vi "main.vi"(0 "Test Pins":T6, 1 "Caller Information":T7, 5 "Test Inputs":T10={"Load Current 1 in A"=0.0, "Load Current 2 in A"=0.0, "Duration of the pulse in Second"=0.5, "Nominal Output Voltage in V"=0.0, "Ref Voltage level for Settling Time Calc"=0.1, "% of Vnom for Settling Time Calc"=10.0, "Settling Time Calc Option"=enum."Voltage Level ", "Advance Setting"={"Prepare"={"Load SMU Record Length"=2}}, "Save Transient Graph?"=TRUE, "Input Voltage in V"=0.0, "Save Scope Raw Data?"=FALSE, "Delay - t1 in s"=0.25, "Delay - t2 in s"=0.25, "Auto Scale Y-Axis?"=TRUE, "Shunt Resistance (Ohm)"=1.0}, 11 "error in":errorcluster) -> (4 "Test Results":T14 {"Second Edge - Settling Time in s" format="%#.5p"; "First Edge - Settling Time in s" format="%#.5p"; "Actual Sample Rate in S/s" format="%#.5g"}, 15 "error out":errorcluster)   [LabVIEW 2020, in "LDO Load Transient.lvlib"]
doc: "<b>Caller</b> Information is input for framework components. Mode should be set to <b>Automation</b> when running from TestStand. Sequence Context should be set to <b>ThisContext</b> when running from TestStand. The values will be updated everytime the setting is applied using \"Edit\" dialog.\n\n<b>Test Pins</b> is names of pins available in the pinmap file. Provide the right pins for the required functionality.\n\n<b>Test Inputs</b> is input required for the measurement to perform.\n\n<b>error in</b> is meant for the sequencing. <b>error in</b> should be <b>no error</b> always.\n\n<b>Test Results</b> contains all the measured data during the measurement and processed results.\n\n<b>error out</b> contains the error occured during measurement.\n\nCheck measurement documentation for more information (<Program Files>\\Soliton Technologies\\MeasurementSuite\\CodeModules\\LDO\\LDO Load Transient.pdf)"
uses:
  LDO Load Transient.lvlib
  Typedefs/Test Results.ctl
  Typedefs/Test Inputs.ctl
  Typedefs/Settling Time Calc Option.ctl
  Typedefs/Advance Settings.ctl
  Typedefs/Adv Settings Setup Instr.ctl
  <userlib>/_Soliton/Measurement Suite/Reusables/Plugin Common/Typedefs/Caller Events.ctl
  <userlib>/_Soliton/Measurement Suite/Reusables/Plugin Common/Typedefs/Caller Information.ctl
  <userlib>/_Soliton/Measurement Suite/Reusables/Plugin Common/Typedefs/Caller Mode.ctl
  Typedefs/Test Pins.ctl
  Typedefs/Pin Dropdown.ctl
  <userlib>/_Soliton/Measurement Suite/Reusables/Plugin Common/Typedefs/Termination Monitor Info.ctl
  Typedefs/Current Measurement Type.ctl
  Reusables/UI/Progress Monitor/Progress Monitor Option.ctl
  <vilib>/Utility/miscctls.llb/LVMajorAndMinorColorsTypeDef.ctl
  <instrlib>/niDCPower/nidcpower.llb/niDCPower Source Mode.ctl
  <instrlib>/niDCPower/nidcpower.llb/niDCPower Output Function.ctl
  <instrlib>/niDCPower/nidcpower.llb/niDCPower Wait For Event - Event.ctl
  <vilib>/Utility/error.llb/DialogType.ctl
  63a61bec-041e-4365-831b-8165c1c311c6.vi
  d648f1df-a8d9-4085-9eb0-24252e83c66e.vi
  98c31a9a-65c4-404a-8d29-5fef3c3d30dc.vi
  feeae9f6-ae23-4438-849e-34acdc15b747.vi
  e89c743e-5273-4ded-a4f4-1d44fefc8133.vi
  44f97677-0516-4608-8e28-d738a12fef77.vi
  01e50ca5-2bbf-454e-9d2d-d5f5dbc62a55.vi
  49732470-67c5-4264-8b59-91d7a6bf13ef.vi
  29f2f23f-c0b0-483c-8177-98a50cbfcdf1.vi
  bb3e62c4-a2c2-4505-9438-f842dd651d6c.vi
  ce2ee1e5-697c-4608-b941-8c9b0f21ffd9.vi
  217e438d-a1ad-49ce-9dcd-d015b5ab8206.vi
  3210b59a-1980-40a2-8b26-190a43568d65.vi
  <userlib>/_Soliton/Measurement Suite/Reusables/InstrumentSessionAPIs/SessionManagerApiPath.vi
  <vilib>/Utility/sysdir.llb/Get System Directory.vi
  <vilib>/Utility/LVLibp/Get Exported File Path.vi
  <userlib>/_Soliton/Measurement Suite/Reusables/Errors/Error 6001.vi
  <userlib>/_Soliton/Measurement Suite/Reusables/Plugin Common/Plugin Common.lvlib
  <userlib>/_Soliton/Measurement Suite/Reusables/Queue Driver/Plugin Queue Driver.lvlib
panel:
  out "Progress":i32(slide) scale=-1.0..17.0
  in  "Terminate":bool
  in  "Run":bool caption="Measure"
  in  "Exit":bool
  out "Header":string
  in  "Tab Enum":T1(radio)
  out "Tab Control":T2(tab)
  in  "Shunt Resistance (Ohm)":dbl=1.0 min=1.0 format="%#_6p"
  in  "SystemSetup":T4={"Set Load Current"={"PinStatus"=0, "PinName"="", "Info"=TRUE}, "Set Input Voltage"={"PinStatus"=0, "PinName"="", "Info"=TRUE}, "Measure Output Voltage"={"PinStatus"=0, "PinName"="", "Info"=TRUE}, "Measure Load Current"={"PinStatus"=0, "PinName"="", "Info"=TRUE}}
  out "Shunt Resistance Info":u16(ring) caption="Set 1 Ohm if its Current Probe"
  out "Sequence Timeout":dbl caption="Sequence Timeout (s)" format="%#.5p"
  in  "Delay - t2 (s)":dbl=0.25 format="%#_6p"
  in  "Delay - t1 (s)":dbl=0.25 format="%#_6p"
  in  "Duration of the pulse (s)":dbl=0.5 format="%#_6p"
  in  "Percentage of Vnom (%)":dbl=10.0 caption="Percentage of nominal voltage (%)" format="%#_6f"
  in  "Voltage to settle above Vnom (V)":dbl=0.1 format="%#_6p"
  in  "Load Current 1 - Iload1 (A)":dbl format="%#_6p"
  in  "Settling Time Calculation":enum32{"Item 0", "Item 1"}(radio)
  in  "Input Voltage (V)":dbl format="%#_6p"
  in  "Load Current 2 - Iload2 (A)":dbl format="%#_6p"
  in  "Nominal Output Voltage (V)":dbl format="%#_6p"
  in  "Advanced Settings":bool
  out "Second Edge - Settling Time (s)":dbl format="%#.5p"
  in  "Auto Scale Y-Axis?":bool=TRUE
  in  "Save Scope Raw Data?":bool=TRUE
  out "Load Transient":cluster{"x-axis":dbl[], "wfm":dbl[]}[](graph)
  in  "Take Transient snapshot?":bool=TRUE
  out "Transient Load Current":waveform(dbl)(graph)
  out "Transient Output Voltage":T5(graph)
  out "First Edge - Settling Time (s)":dbl format="%#.5p"
  in  "Caller Events":T9
  in  "DataLogPath":path
  in  "ErrorOccured":errorcluster
  # "Supports NIDCPowerInstrument"
  # "Supports NIScopeInstrument"
  # "Supports NIDCPowerInstrument"
  # "Supports NIScopeInstrument,NIDCPowerInstrument"
  # "Load Current"
  # "Minimum value for Delay-t1, Duration of the pulse, Delay-t2 should be larger than [ ( Souredelay+Aperture Time ) x Record Length ]"
  # "Settling Time Calculation"
  # "Settling Time is defined as the time taken for the output voltage to recover\nto the LDO nominal output voltage."
  # "Time taken for output voltage to settle to (Choose one below)"
  # "Load Transient"
  # "Output Voltage"
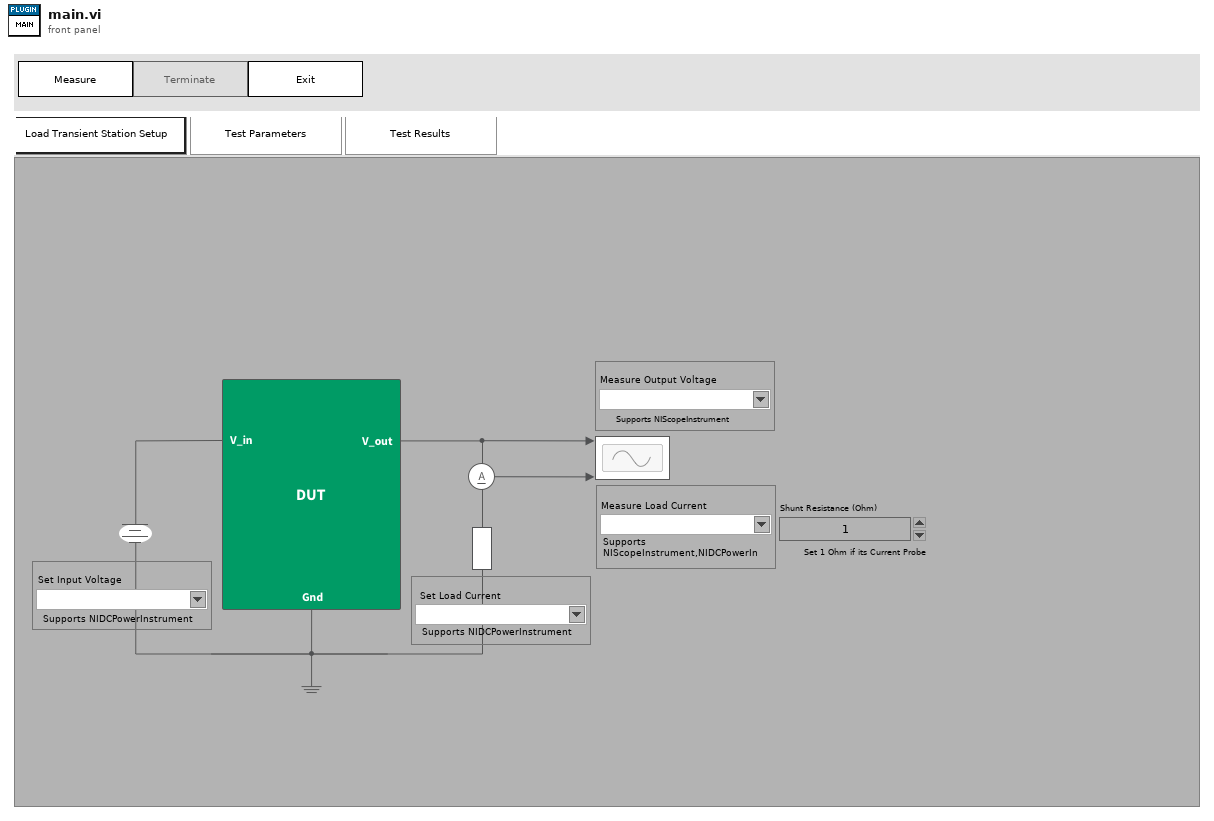
[diagram p1: front panel]
types:
  T1 = enum32{"Station Setup", "Test Parameters", "Test Results"}
  T2 = enum32{"Station Setup", "Test Parameters", "Test Results", "Debug"}
  T3 = typedef "LDO Load Transient.lvlib/Pin Dropdown.ctl" = cluster{"PinStatus":u16, "PinName":string, "Info":bool}
  T4 = cluster{"Set Load Current":T3, "Set Input Voltage":T3, "Measure Output Voltage":T3, "Measure Load Current":T3}
  T5 = cluster{"relativeInitialX":dbl, "xIncrement":dbl, "wfm":dbl[]}
  T6 = typedef "LDO Load Transient.lvlib/Test Pins.ctl" = cluster{"Set Input Voltage":string, "Set Load Current":string, "Measure Output Voltage":string, "Measure Load Current":string}
  T7 = typedef "Plugin Common.lvlib/Caller Information.ctl" = cluster{"Mode":T8, "Sequence Context":refnum<k7>}
  T8 = typedef "Caller Mode.ctl" = enum16{"Standalone", "Automation", "MeasurementSuite"}
  T9 = typedef "Plugin Common.lvlib/Caller Events.ctl" = cluster{"Caller Event":refnum<user-event>}
  T10 = typedef "LDO Load Transient.lvlib/Test Inputs.ctl" = cluster{"Load Current 1 in A":dbl, "Load Current 2 in A":dbl, "Duration of the pulse in Second":dbl, "Nominal Output Voltage in V":dbl, "Ref Voltage level for Settling Time Calc":dbl, "% of Vnom for Settling Time Calc":dbl, "Settling Time Calc Option":T11, "Advance Setting":T12, "Save Transient Graph?":bool, "Input Voltage in V":dbl, "Save Scope Raw Data?":bool, "Delay - t1 in s":dbl, "Delay - t2 in s":dbl, "Auto Scale Y-Axis?":bool, "Shunt Resistance (Ohm)":dbl}
  T11 = typedef "LDO Load Transient.lvlib/Settling Time Calc Option.ctl" = enum16{"Voltage Level ", "Percentage of Vnom"}
  T12 = typedef "LDO Load Transient.lvlib/Advance Settings.ctl" = cluster{"Prepare":T13}
  T13 = typedef "LDO Load Transient.lvlib/Adv Settings Setup Instr.ctl" = cluster{"Load SMU Record Length":i32}
  T14 = typedef "LDO Load Transient.lvlib/Test Results.ctl" = cluster{"Measured Output Voltage":cluster{"x-axis":dbl[], "wfm":dbl[]}, "Measured Load Current":cluster{"x-axis":dbl[], "wfm":dbl[]}, "Actual Sample Rate in S/s":dbl, "First Edge - Settling Time in s":dbl, "Second Edge - Settling Time in s":dbl}
  T15 = typedef "Plugin Common.lvlib/Termination Monitor Info.ctl" = cluster{"Caller Information":T7, "Execution":refnum<k7>, "Termination Monitor":refnum<k7>, "Type":string, "Plugin Name":string}
  T16 = typedef "LDO Load Transient.lvlib/Current Measurement Type.ctl" = enum16{"Scope Measurement", "SMU Measurement"}
  T17 = cluster{"Termination Monitor Info":T15, "Test Inputs":T10, "Test Results":T14, "Test Results[][]":string[][], "Test Pins":T6, "Logger Folder Path":path, "Valid Logger Path?":bool, "Logger File Path":path, "Load Current Waveform":dbl[], "Load Current Source Delay":dbl[], "Min delay for Reference Position":u32, "Output Voltage Coupling":i32, "Current Measurement Option":T16, "Sequence name":string, "UI Ctls":refnum<vi>[], "Insufficient memory?":bool, "Scope Record Length":i32, "Scope Channels":string, "Sequence Empty?":bool}
  T18 = typedef "Progress Monitor Option.ctl" = enum16{"State Array Init", "Get State Index"}
  T19 = enum8{"Enabled", "Disabled", "Disabled and Grayed Out"}
  T20 = cluster{"Set Iload":T3, "Set Vin":T3, "Capture Output Voltage":T3, "Capture Output Current":T3}
  T21 = typedef "LVMajorAndMinorColorsTypeDef.ctl" = cluster{"Major Color":u32, "Minor Color":u32}
  T22 = typedef "niDCPower Wait For Event - Event.ctl" = i32
  T23 = typedef "niDCPower Output Function.ctl" = i32
  T24 = typedef "niDCPower Source Mode.ctl" = i32
  T25 = typedef "DialogType.ctl" = u16
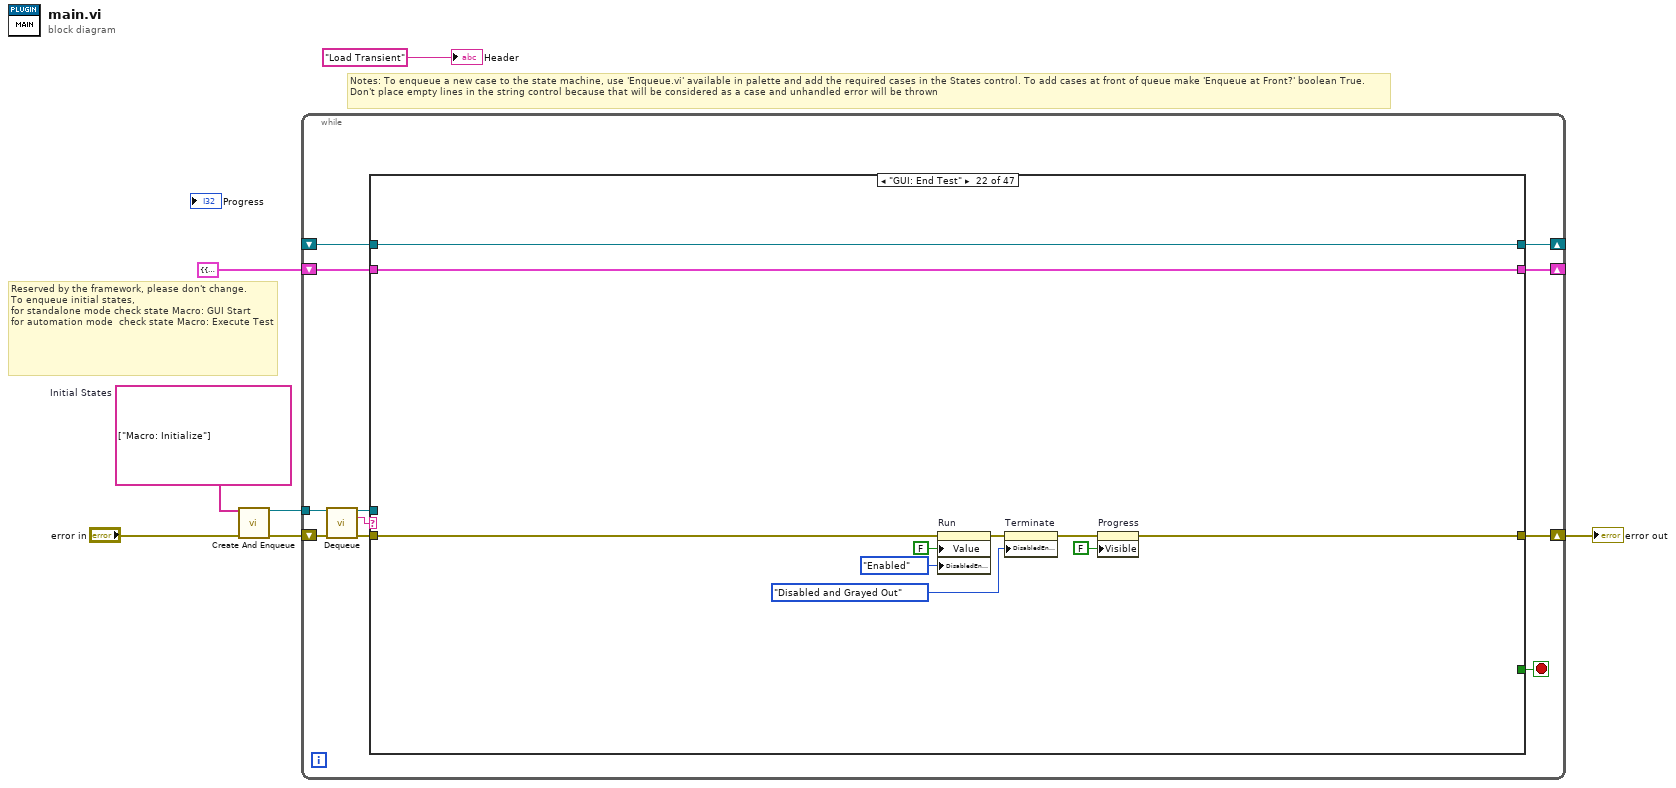
[diagram p0: block diagram]
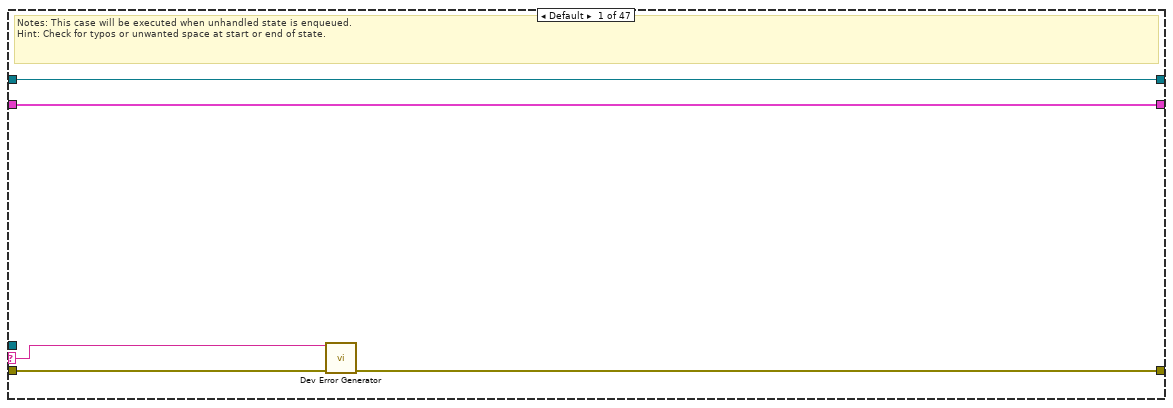
[diagram p2: hidden frame]
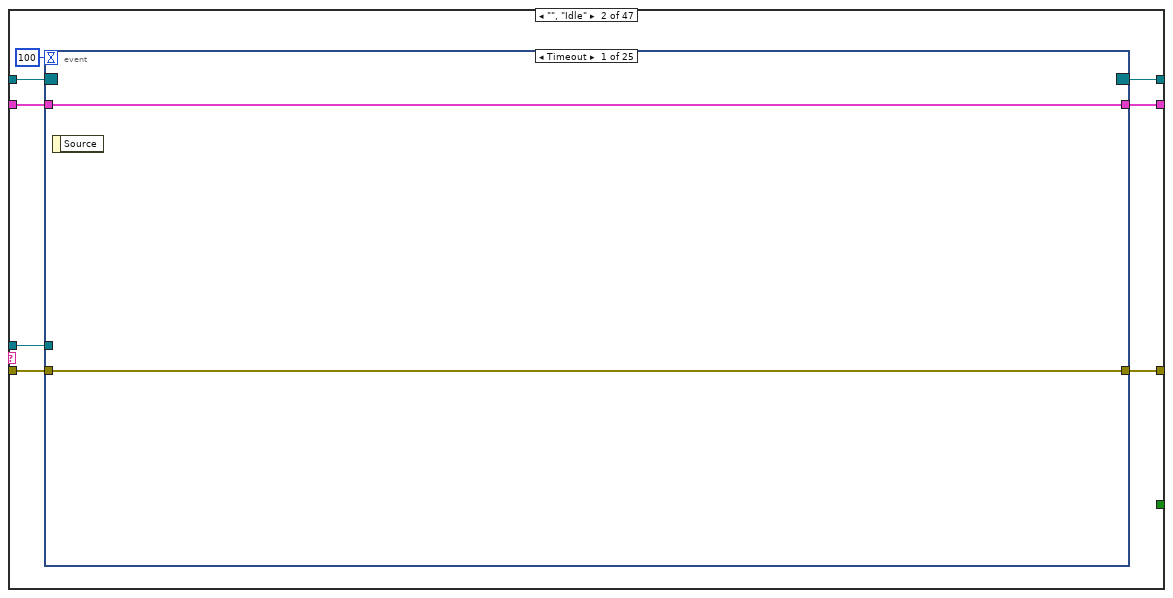
[diagram p3: hidden frame]
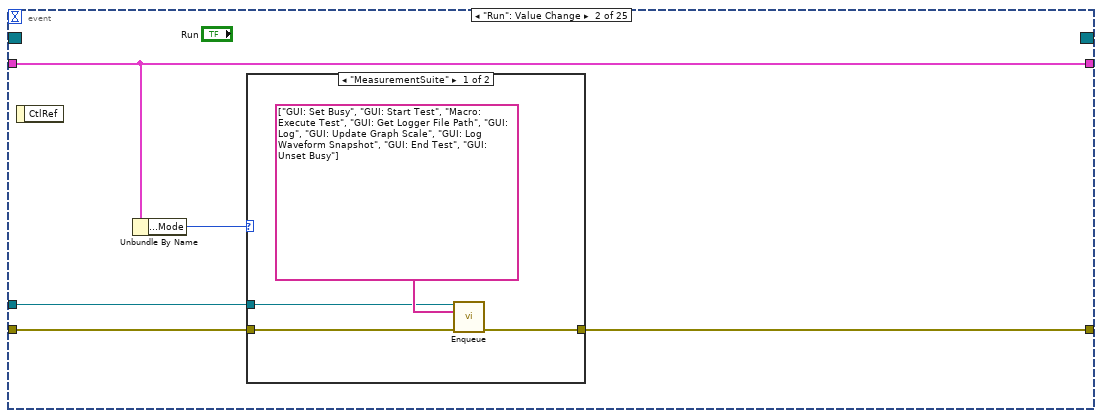
[diagram p4: hidden frame]
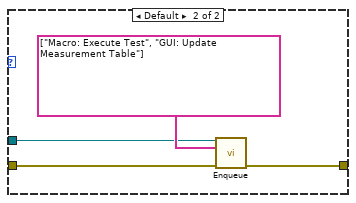
[diagram p5: hidden frame]
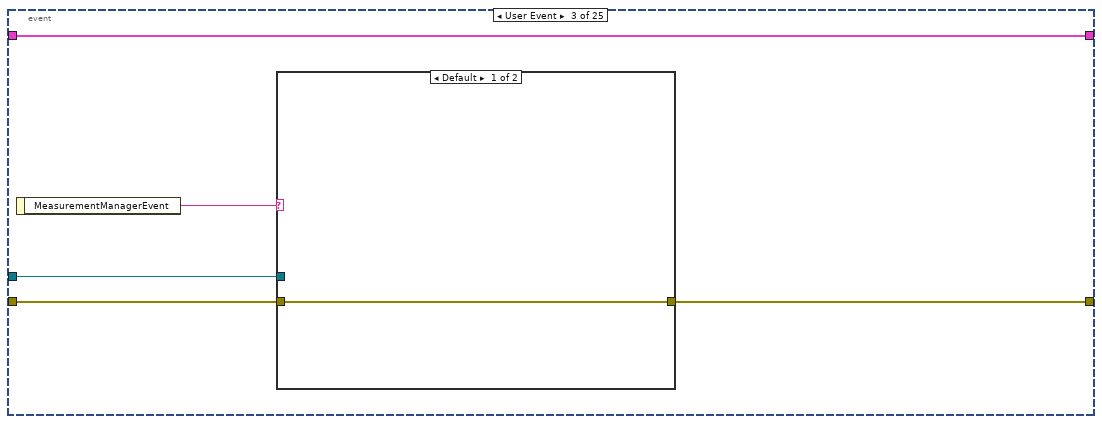
[diagram p6: hidden frame]
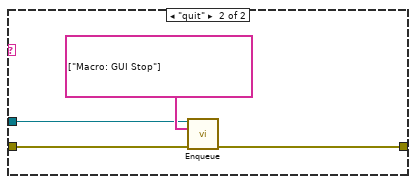
[diagram p7: hidden frame]
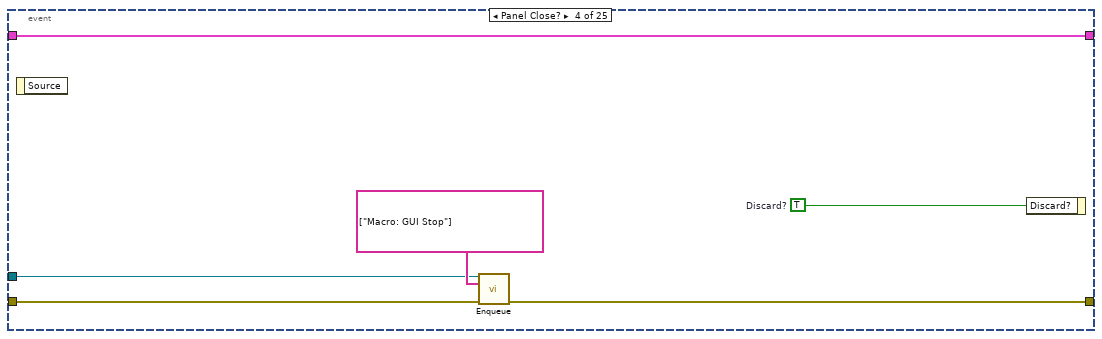
[diagram p8: hidden frame]
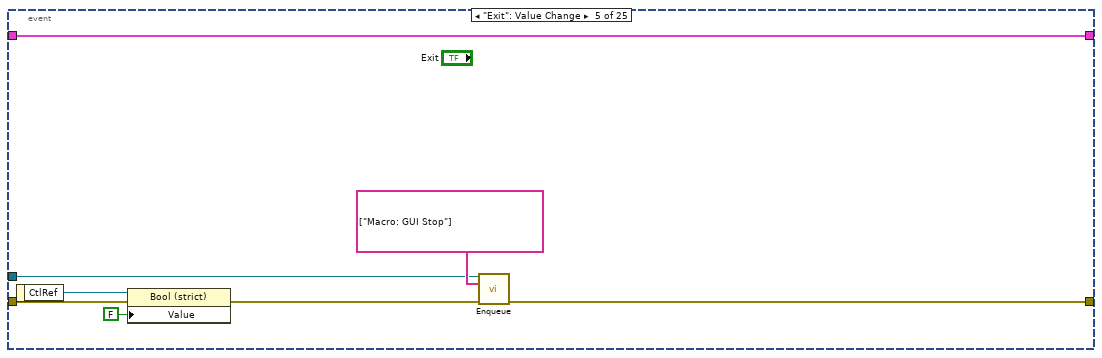
[diagram p9: hidden frame]
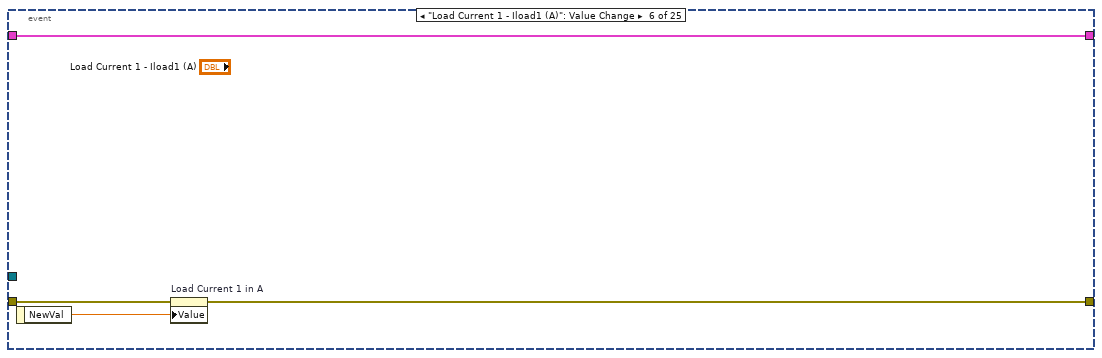
[diagram p10: hidden frame]
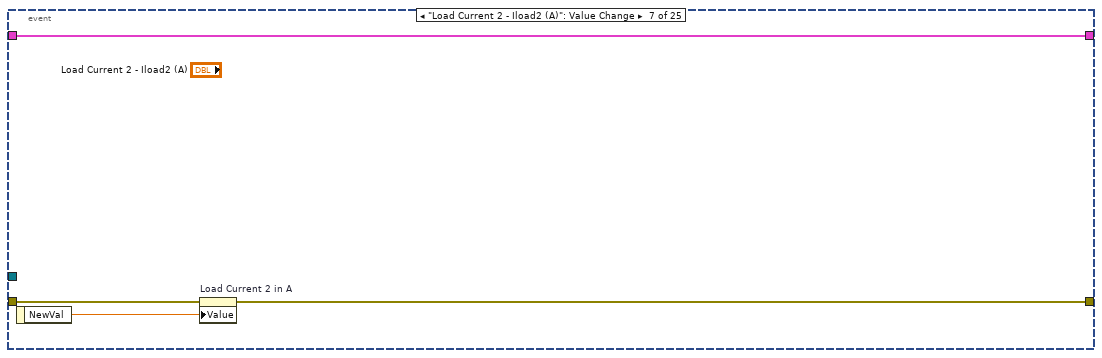
[diagram p11: hidden frame]
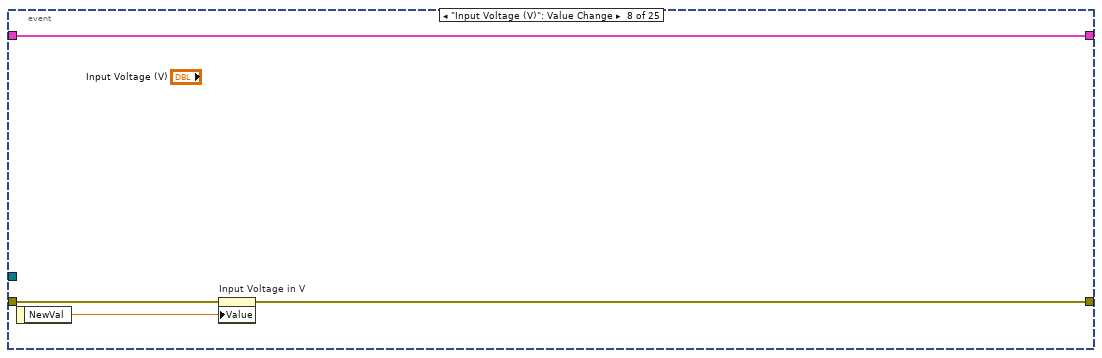
[diagram p12: hidden frame]
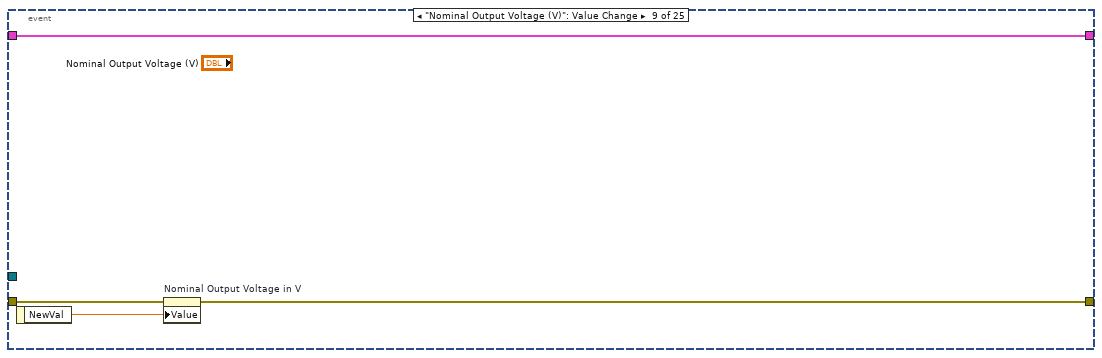
[diagram p13: hidden frame]
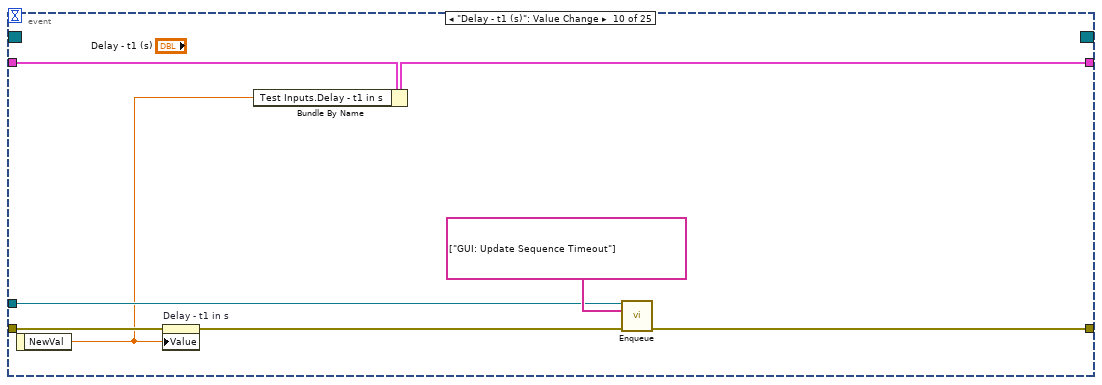
[diagram p14: hidden frame]
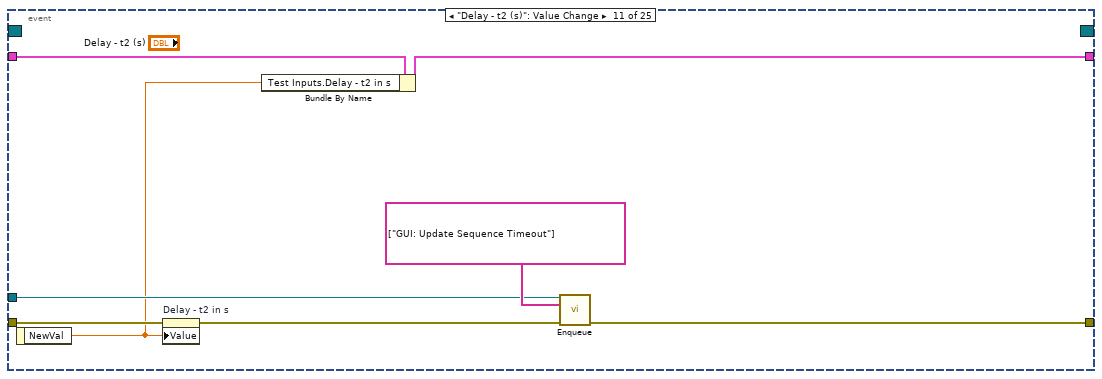
[diagram p15: hidden frame]
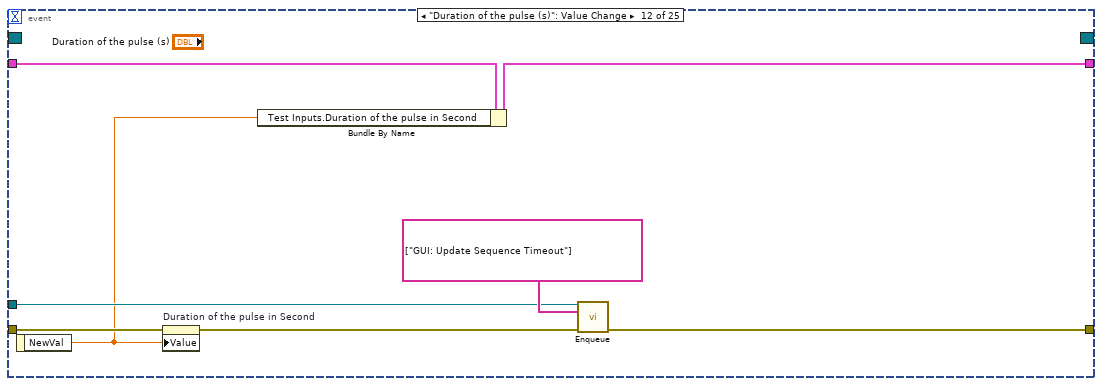
[diagram p16: hidden frame]
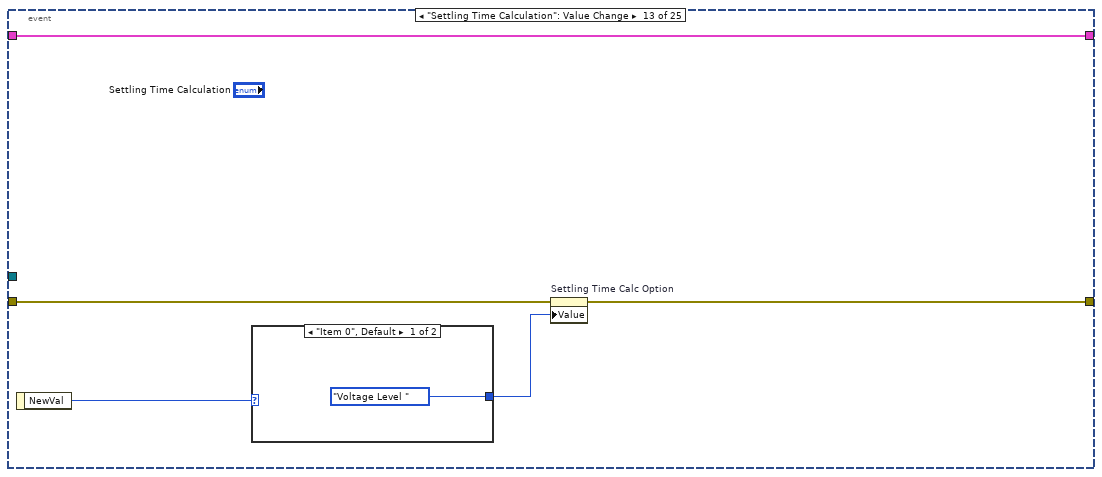
[diagram p17: hidden frame]
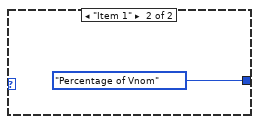
[diagram p18: hidden frame]
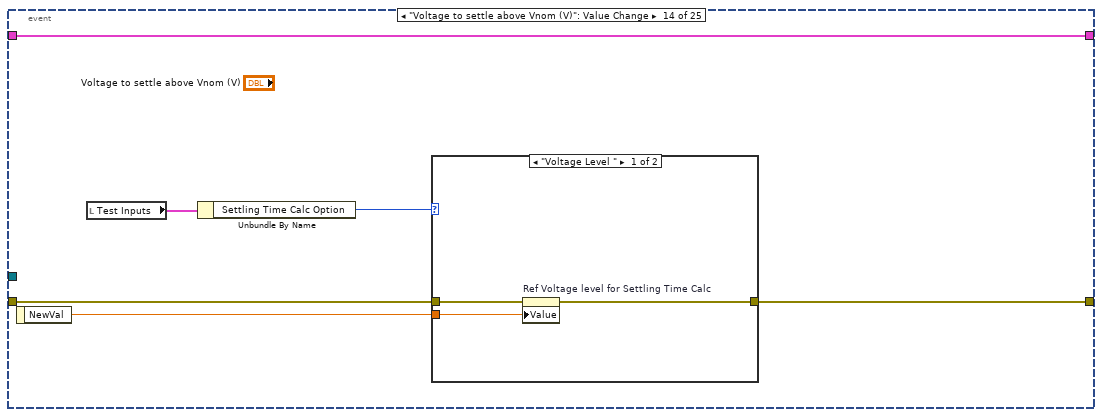
[diagram p19: hidden frame]
diagram:
  w7 = string[] ["Macro: Initialize"]  # Initial States
  # "Notes: To enqueue a new case to the state machine, use 'Enqueue.vi' available in palette and add the required cases in the States control. To add cases at front of queue make 'Enqueue at Front?' boolean True. Don't place empty lines in the string control because that will be considered as a case and unhandled error will be thrown"
  # "Reserved by the framework, please don't change. \nTo enqueue initial states,\nfor standalone mode check state Macro: GUI Start\nfor automation mode  check state Macro: Execute Test"
  n1 = call <userlib>:"Create And Enqueue.vi"("Initial States"=w7, "error in (no error)"="error in") -> ("Queue out"=w5:refnum<queue>, "error out"=w3:errorcluster)  [unwired: 12 in]
  n2 = while {
    shift-right: [w18] -> w4
    shift-left: w3 -> [w16]
    shift-right: [w14] -> _
    shift-left: T17 {"Termination Monitor Info"={"Caller Information"={"Mode"=enum."Standalone", "Sequence Context"=refnum}, "Execution"=refnum, "Termination Monitor"=refnum, "Type"="", "Plugin Name"=""}, "Test Inputs"={"Load Current 1 in A"=0.0, "Load Current 2 in A"=0.0, "Duration of the pulse in Second"=0.0, "Nominal Output Voltage in V"=0.0, "Ref Voltage level for Settling Time Calc"=0.0, "% of Vnom for Settling Time Calc"=0.0, "Settling Time Calc Option"=enum."Voltage Level ", "Advance Setting"={"Prepare"={"Load SMU Record Length"=0}}, "Save Transient Graph?"=FALSE, "Input Voltage in V"=0.0, "Save Scope Raw Data?"=FALSE, "Delay - t1 in s"=0.0, "Delay - t2 in s"=0.0, "Auto Scale Y-Axis?"=FALSE, "Shunt Resistance (Ohm)"=0.0}, "Test Results"={"Measured Output Voltage"={"x-axis"=[], "wfm"=[]}, "Measured Load Current"={"x-axis"=[], "wfm"=[]}, "Actual Sample Rate in S/s"=0.0, "First Edge - Settling Time in s"=0.0, "Second Edge - Settling Time in s"=0.0}, "Test Results[][]"=[], "Test Pins"={"Set Input Voltage"="", "Set Load Current"="", "Measure Output Voltage"="", "Measure Load Current"=""}, "Logger Folder Path"=path "", "Valid Logger Path?"=FALSE, "Logger File Path"=path "", "Load Current Waveform"=[], "Load Current Source Delay"=[], "Min delay for Reference Position"=0, "Output Voltage Coupling"=0, "Current Measurement Option"=enum."Scope Measurement", "Sequence name"="CurrentSequence", "UI Ctls"=[], "Insufficient memory?"=FALSE, "Scope Record Length"=0, "Scope Channels"="", "Sequence Empty?"=TRUE} -> [w13]
    tunnel: w5 -> [w12]
    shift-right: [w9] -> _
    shift-left: _ -> [w10]
    stop <- w17 stop-if-true
    n3 = call <userlib>:"Dequeue.vi"("Queue in"=w12, "error in (no error)"=w16) -> ("Queue out"=w11:refnum<queue>, "Dequeued State"=w8:string, "error out"=w15:errorcluster)  [unwired: 11 in]
    n4 = case shown="\"GUI: End Test\"" w8 {
      selector: w8 -> [w21 _ _ _ _ _ _ _ _ _ _ _ w345 w361 _ _ _ _ _ _ _ _ _ _ _ _ w537 w554 w567 w602 w630 w675 _ _ w746 w755 w795 w834 w867 w883 w928 w955 w981 w990 _ _ _]
      tunnel: w15 -> [w20 w28 w251 w260 w275 w281 w288 w293 w326 w337 w341 w344 w346 w363 w378 w391 w403 w432 w445 w466 w498 w507 w518 w523 w530 w535 w538 w555 w568 w603 w631 w676 w692 w706 w747 w756 w796 w835 w868 w884 w929 w956 w982 w991 w998 w1005 w1023]
      tunnel: [w22 w29 w251 w263 w266 w282 w289 w293 w324 w335 w339 w344 w350 w366 w379 w392 w402 w433 w443 w467 w499 w506 w518 w524 w531 w535 w544 w561 w566 w584 w634 w683 w693 w707 w745 w763 w790 w829 w869 w885 w915 w959 w983 w992 w998 w1003 w1017] -> w18
      tunnel: [_ _ _ _ _ _ _ _ _ _ _ _ _ _ _ _ _ _ _ _ _ _ _ _ _ _ _ _ _ _ _ _ _ _ _ _ _ _ _ _ _ _ _ _ _ w1000 TRUE] -> w17
      tunnel: [w23 w31 w250 w253 w276 w283 w290 w292 w315 w336 w340 w343 w349 w365 w380 w398 w401 w434 w459 w465 w505 w515 w517 w522 w529 w534 w543 w560 w571 w608 w629 w681 w691 w709 w750 w760 w798 w838 w872 w888 w936 w961 w988 w995 w997 w1002 w1024] -> w14
      tunnel: w13 -> [w23 w30 w250 w264 w276 w283 w290 w292 w331 w336 w340 w343 w349 w365 w380 w398 w400 w434 w459 w465 w505 w515 w517 w521 w528 w534 w553 w559 w571 w608 w628 w680 w690 w708 w750 w759 w798 w837 w871 w887 w936 w961 w988 w995 w997 w1002 w1024]
      tunnel: w11 -> [_ w24 _ w262 w274 w279 w286 _ _ _ _ _ _ _ _ _ _ _ _ _ _ _ _ _ _ _ _ _ _ _ _ _ _ _ _ _ _ _ _ _ _ _ _ _ _ w999 w1022]
      tunnel: w10 -> [w19 w26 w249 w261 w273 w278 w285 w291 w330 _ w338 w342 w356 w372 w381 w399 w408 w435 w460 w472 w504 w514 w516 w525 w532 w533 w551 w563 w572 w609 w636 w688 w695 w711 w751 w764 w799 w839 w878 w897 w937 w966 w989 w994 w996 w1004 w1021]
      tunnel: [w19 w25 w249 w261 w273 w278 w285 w291 w330 w334 w338 w342 w356 w372 w381 w399 w408 w435 w460 w472 w504 w514 w516 w525 w532 w533 w551 w563 w572 w609 w636 w688 w695 w711 w751 w764 w799 w839 w878 w897 w937 w966 w989 w994 w996 w1004 w1021] -> w9
      frame Default {
        # "Notes: This case will be executed when unhandled state is enqueued. \nHint: Check for typos or unwanted space at start or end of state."
        n5 = call <userlib>:"Dev Error Generator.vi"("State"=w21, "error in (no error)"=w20) -> ("error out"=w22:errorcluster)  [unwired: 13 in]
      }
      frame "", "Idle" {
        n6 = event shown="[0] Timeout" {
          selector: w26 -> [_ _ _ _ _ _ _ _ _ _ _ _ _ _ _ _ _ _ _ _ _ _ _ _ _]
          dyn-events: [_ _ _ _ _ _ _ _ _ _ _ _ _ _ _ _ _ _ _ _ _ _ _ _ _] -> w25
          timeout: 100 -> [_ _ _ _ _ _ _ _ _ _ _ _ _ _ _ _ _ _ _ _ _ _ _ _ _]
          tunnel: [w33 w35 w51 w62 w70 w74 w78 w82 w86 w89 w97 w105 w115 w123 w134 w145 w149 w153 w158 w169 w188 w232 w237 w242 w248] -> w31
          tunnel: w30 -> [w33 w35 w51 w62 w70 w74 w78 w82 w86 w88 w96 w104 w115 w123 w134 w145 w149 w153 w160 w168 w187 w231 w237 w241 w248]
          tunnel: [w32 w38 w49 w59 w68 w73 w77 w80 w85 w91 w99 w107 w112 w121 w131 w143 w147 w151 w154 w167 w179 w213 w236 w239 w246] -> w29
          tunnel: w28 -> [w32 w37 w50 w58 w67 w72 w76 w81 w84 w94 w102 w110 w113 w122 w130 w144 w148 w152 w159 w170 w190 w212 w236 w244 w247]
          tunnel: w24 -> [_ w36 w47 w57 w66 _ _ _ _ w90 w98 w106 _ _ _ _ _ _ _ w166 w178 _ _ _ _]
          event Timeout {
            n7 = event-data() -> ()  [unwired: 1 in, 1 out]
          }
          event "Run": Value Change {
            n8 = event-data() -> ()  [unwired: 1 in, 1 out]
            n9 = Unbundle By Name(w35) -> ("Termination Monitor Info.Caller Information.Mode"=w34:T8)
            n10 = case shown="\"MeasurementSuite\"" w34 {
              tunnel: [w41 w45] -> w38
              tunnel: w37 -> [w40 w44]
              tunnel: w36 -> [w39 w43]
              frame "MeasurementSuite" {
                n11 = call <userlib>:"Enqueue.vi"("Queue in"=w39, "States"=string[] ["GUI: Set Busy", "GUI: Start Test", "Macro: Execute Test", "GUI: Get Logger File Path", "GUI: Log", "GUI: Update Graph Scale", "GUI: Log Waveform Snapshot", "GUI: End Test", "GUI: Unset Busy"], "error in (no error)"=w40) -> ("error out"=w41:errorcluster)  [unwired: 11 in, 1 out]
              }
              frame Default {
                n12 = call <userlib>:"Enqueue.vi"("Queue in"=w43, "States"=string[] ["Macro: Execute Test", "GUI: Update Measurement Table"], "error in (no error)"=w44) -> ("error out"=w45:errorcluster)  [unwired: 11 in, 1 out]
              }
            }
          }
          event User Event {
            n13 = event-data() -> ("MeasurementManagerEvent"=w48:string)  [unwired: 1 in]
            n14 = case shown="Default" w48 {
              tunnel: [w52 w53] -> w49
              tunnel: w50 -> [w52 w55]
              tunnel: w47 -> [_ w54]
              frame Default {
              }
              frame "quit" {
                n15 = call <userlib>:"Enqueue.vi"("Queue in"=w54, "States"=string[] ["Macro: GUI Stop"], "error in (no error)"=w55) -> ("error out"=w53:errorcluster)  [unwired: 11 in, 1 out]
              }
            }
          }
          event Panel Close? {
            w61 = TRUE  # Discard?
            n16 = event-data() -> ()  [unwired: 1 in, 1 out]
            n17 = call <userlib>:"Enqueue.vi"("Queue in"=w57, "States"=string[] ["Macro: GUI Stop"], "error in (no error)"=w58) -> ("error out"=w59:errorcluster)  [unwired: 11 in, 1 out]
            n18 = event-data("Discard?"=w61) -> ()  [unwired: 1 in, 1 out]
          }
          event "Exit": Value Change {
            n19 = event-data() -> ("CtlRef"=w64:refnum<vi>)  [unwired: 1 in]
            n20 = property class="Bool (strict)"(reference=w64, error in=w67, "Value"=FALSE) -> (error out=w65:errorcluster)  [unwired: 1 out]
            n21 = call <userlib>:"Enqueue.vi"("Queue in"=w66, "States"=string[] ["Macro: GUI Stop"], "error in (no error)"=w65) -> ("error out"=w68:errorcluster)  [unwired: 11 in, 1 out]
          }
          event "Load Current 1 - Iload1 (A)": Value Change {
            n22 = event-data() -> ("NewVal"=w71:dbl)  [unwired: 1 in]
            n23 = property on="Load Current 1 in A" class="DigNum (strict)"(error in=w72, "Value"=w71) -> (error out=w73:errorcluster)  [unwired: 1 in, 1 out]
          }
          event "Load Current 2 - Iload2 (A)": Value Change {
            n24 = event-data() -> ("NewVal"=w75:dbl)  [unwired: 1 in]
            n25 = property on="Load Current 2 in A" class="DigNum (strict)"(error in=w76, "Value"=w75) -> (error out=w77:errorcluster)  [unwired: 1 in, 1 out]
          }
          event "Input Voltage (V)": Value Change {
            n26 = event-data() -> ("NewVal"=w79:dbl)  [unwired: 1 in]
            n27 = property on="Input Voltage in V" class="DigNum (strict)"(error in=w81, "Value"=w79) -> (error out=w80:errorcluster)  [unwired: 1 in, 1 out]
          }
          event "Nominal Output Voltage (V)": Value Change {
            n28 = event-data() -> ("NewVal"=w83:dbl)  [unwired: 1 in]
            n29 = property on="Nominal Output Voltage in V" class="DigNum (strict)"(error in=w84, "Value"=w83) -> (error out=w85:errorcluster)  [unwired: 1 in, 1 out]
          }
          event "Delay - t1 (s)": Value Change {
            n30 = event-data() -> ("NewVal"=w87:dbl)  [unwired: 1 in]
            n31 = property on="Delay - t1 in s" class="DigNum (strict)"(error in=w94, "Value"=w87) -> (error out=w92:errorcluster)  [unwired: 1 in, 1 out]
            n32 = Bundle By Name(cluster=w88, "Test Inputs.Delay - t1 in s"=w87) -> (w89:T17)
            n33 = call <userlib>:"Enqueue.vi"("Queue in"=w90, "States"=string[] ["GUI: Update Sequence Timeout"], "error in (no error)"=w92) -> ("error out"=w91:errorcluster)  [unwired: 11 in, 1 out]
          }
          event "Delay - t2 (s)": Value Change {
            n34 = event-data() -> ("NewVal"=w95:dbl)  [unwired: 1 in]
            n35 = property on="Delay - t2 in s" class="DigNum (strict)"(error in=w102, "Value"=w95) -> (error out=w100:errorcluster)  [unwired: 1 in, 1 out]
            n36 = Bundle By Name(cluster=w96, "Test Inputs.Delay - t2 in s"=w95) -> (w97:T17)
            n37 = call <userlib>:"Enqueue.vi"("Queue in"=w98, "States"=string[] ["GUI: Update Sequence Timeout"], "error in (no error)"=w100) -> ("error out"=w99:errorcluster)  [unwired: 11 in, 1 out]
          }
          event "Duration of the pulse (s)": Value Change {
            n38 = event-data() -> ("NewVal"=w103:dbl)  [unwired: 1 in]
            n39 = property on="Duration of the pulse in Second" class="DigNum (strict)"(error in=w110, "Value"=w103) -> (error out=w108:errorcluster)  [unwired: 1 in, 1 out]
            n40 = Bundle By Name(cluster=w104, "Test Inputs.Duration of the pulse in Second"=w103) -> (w105:T17)
            n41 = call <userlib>:"Enqueue.vi"("Queue in"=w106, "States"=string[] ["GUI: Update Sequence Timeout"], "error in (no error)"=w108) -> ("error out"=w107:errorcluster)  [unwired: 11 in, 1 out]
          }
          event "Settling Time Calculation": Value Change {
            n42 = event-data() -> ("NewVal"=w114:enum32{"Item 0", "Item 1"})  [unwired: 1 in]
            n43 = case shown="\"Item 0\", Default" w114 {
              tunnel: [Settling_Time_Calc_Option."Voltage Level " ("Value") Settling_Time_Calc_Option."Percentage of Vnom" ("Value")] -> w111
              frame "Item 0", Default {
              }
              frame "Item 1" {
              }
            }
            n44 = property on="Settling Time Calc Option" class="Enum (strict)"(error in=w113, "Value"=w111) -> (error out=w112:errorcluster)  [unwired: 1 in, 1 out]
          }
          event "Voltage to settle above Vnom (V)": Value Change {
            n45 = event-data() -> ("NewVal"=w118:dbl)  [unwired: 1 in]
            n46 = local read "Test Inputs"() -> (w120:T10)
            n47 = Unbundle By Name(w120) -> ("Settling Time Calc Option"=w119:T11)
            n48 = case shown="\"Voltage Level \"" w119 {
              tunnel: w122 -> [w126 w127]
              tunnel: [w125 w127] -> w121
              tunnel: w118 -> [w124 _]
              frame "Voltage Level " {
                n49 = property on="Ref Voltage level for Settling Time Calc" class="DigNum (strict)"(error in=w126, "Value"=w124) -> (error out=w125:errorcluster)  [unwired: 1 in, 1 out]
              }
              frame "Percentage of Vnom", Default {
              }
            }
          }
          event "Percentage of Vnom (%)": Value Change {
            n50 = event-data() -> ("NewVal"=w129:dbl)  [unwired: 1 in]
            n51 = local read "Test Inputs"() -> (w132:T10)
            n52 = Unbundle By Name(w132) -> ("Settling Time Calc Option"=w133:T11, "Nominal Output Voltage in V"=w128:dbl)
            n53 = case shown="\"Percentage of Vnom\"" w133 {
              tunnel: w130 -> [w135 w141]
              tunnel: [w135 w137] -> w131
              tunnel: w129 -> [_ w136]
              tunnel: w128 -> [_ w138]
              frame "Voltage Level ", Default {
              }
              frame "Percentage of Vnom" {
                n54 = formula code="y = (x/100)*v;"("v"=w138, "x"=w136) -> ("y"=w139:dbl)
                n55 = property on="Ref Voltage level for Settling Time Calc" class="DigNum (strict)"(error in=w141, "Value"=w139) -> (error out=w140:errorcluster)  [unwired: 1 in, 1 out]
                n56 = property on="% of Vnom for Settling Time Calc" class="DigNum (strict)"(error in=w140, "Value"=w136) -> (error out=w137:errorcluster)  [unwired: 1 in, 1 out]
              }
            }
          }
          event "Take Transient snapshot?": Value Change {
            n57 = event-data() -> ("NewVal"=w142:bool)  [unwired: 1 in]
            n58 = property on="Save Transient Graph?" class="Bool (strict)"(error in=w144, "Value"=w142) -> (error out=w143:errorcluster)  [unwired: 1 in, 1 out]
          }
          event "Save Scope Raw Data?": Value Change {
            n59 = event-data() -> ("NewVal"=w146:bool)  [unwired: 1 in]
            n60 = property on="Save Scope Raw Data?" class="Bool (strict)"(error in=w148, "Value"=w146) -> (error out=w147:errorcluster)  [unwired: 1 in, 1 out]
          }
          event "Auto Scale Y-Axis?": Value Change {
            n61 = event-data() -> ("NewVal"=w150:bool)  [unwired: 1 in]
            n62 = property on="Auto Scale Y-Axis?" class="Bool (strict)"(error in=w152, "Value"=w150) -> (error out=w151:errorcluster)  [unwired: 1 in, 1 out]
          }
          event "SystemSetup": Value Change {
            n63 = event-data() -> ("NewVal"=w155:T4)  [unwired: 1 in]
            n64 = Unbundle By Name(w155) -> ("Set Input Voltage.PinName"=w163:string, "Set Load Current.PinName"=w162:string, "Measure Output Voltage.PinName"=w161:string, "Measure Load Current.PinName"=w156:string)
            n65 = Bundle By Name(cluster=w160, "Test Pins.Set Input Voltage"=w163, "Test Pins.Set Load Current"=w162, "Test Pins.Measure Output Voltage"=w161, "Test Pins.Measure Load Current"=w156) -> (w158:T17)
            n66 = Unbundle By Name(w158) -> ("Test Pins"=w157:T6)
            n67 = property on="Test Pins" class="Clust (strict)"(error in=w159, "Value"=w157) -> (error out=w154:errorcluster)  [unwired: 1 in, 1 out]
          }
          event Value Change {
            n68 = event-data() -> ("NewVal.PinName"=w165:string)  [unwired: 1 in]
            n69 = Bundle By Name(cluster=w168, "Test Pins.Measure Load Current"=w165) -> (w169:T17)
            n70 = Empty String/Path?(string/path=w165) -> (empty?=w164:bool)
            n71 = case shown="True" w164 {
              tunnel: w170 -> [w174 w175]
              tunnel: [w172 w175] -> w167
              tunnel: w166 -> [w171 _]
              frame False {
                # "Update Current Measurement option and Shunt Resistance"
                n72 = call <userlib>:"Enqueue.vi"("Queue in"=w171, "States"=string[] ["Test: Get Current Measurement Option", "GUI: Update Shunt Resistance Display"], "error in (no error)"=w174) -> ("error out"=w172:errorcluster)  [unwired: 11 in, 1 out]
              }
              frame True {
              }
            }
          }
          event Value Change {
            n73 = event-data() -> ("NewVal"=w176:T6, "NewVal.Set Input Voltage"=w186:string, "NewVal.Set Load Current"=w185:string, "NewVal.Measure Output Voltage"=w184:string, "NewVal.Measure Load Current"=w177:string)  [unwired: 1 in]
            n74 = Bundle By Name(cluster=w187, "Test Pins"=w176) -> (w188:T17)
            n75 = property on="SystemSetup" class="Clust (strict)"(error in=w190) -> (error out=w189:errorcluster, "Value"=w183:T20)  [unwired: 1 in, 1 out]
            n76 = Bundle By Name(cluster=w183, "Set Vin.PinName"=w186, "Set Iload.PinName"=w185, "Capture Output Voltage.PinName"=w184, "Capture Output Current.PinName"=w177) -> (w182:T20)
            n77 = property on="SystemSetup" class="Clust (strict)"(error in=w189, "Value"=w182) -> (error out=w180:errorcluster)  [unwired: 1 in, 1 out]
            n78 = Empty String/Path?(string/path=w177) -> (empty?=w181:bool)
            n79 = case shown="False" w181 {
              tunnel: w180 -> [w194 w195]
              tunnel: [w192 w195] -> w179
              tunnel: w178 -> [w191 _]
              frame False {
                # "Update Current Measurement option and Shunt Resistance"
                n80 = call <userlib>:"Enqueue.vi"("Queue in"=w191, "States"=string[] ["Test: Get Current Measurement Option", "GUI: Update Shunt Resistance Display"], "error in (no error)"=w194) -> ("error out"=w192:errorcluster)  [unwired: 11 in, 1 out]
              }
              frame True {
              }
            }
          }
          event Value Change {
            n81 = event-data() -> ("NewVal.Advance Setting"=w233:T12, "NewVal.Load Current 1 in A"=w225:dbl, "NewVal.Load Current 2 in A"=w224:dbl, "NewVal.Input Voltage in V"=w223:dbl, "NewVal.Nominal Output Voltage in V"=w222:dbl, "NewVal.Ref Voltage level for Settling Time Calc"=w221:dbl, "NewVal.% of Vnom for Settling Time Calc"=w220:dbl, "NewVal.Settling Time Calc Option"=w219:T11, "NewVal.Save Transient Graph?"=w215:bool, "NewVal.Delay - t1 in s"=w199:dbl, "NewVal.Delay - t2 in s"=w200:dbl, "NewVal.Duration of the pulse in Second"=w201:dbl, "NewVal.Save Scope Raw Data?"=w207:bool, "NewVal.Auto Scale Y-Axis?"=w206:bool, "NewVal.Shunt Resistance (Ohm)"=w204:dbl)  [unwired: 1 in]
            n82 = property on="Input \nVoltage 1 \n- Vin1 (V)" class="DigNum (strict)"(error in=w212, "Value"=w225) -> (error out=w226:errorcluster)  [unwired: 1 in, 1 out]
            n83 = property on="Delay - t1 (s)" class="DigNum (strict)"(error in=w212, "Value"=w199) -> (error out=w209:errorcluster)  [unwired: 1 in, 1 out]
            n84 = property on="Delay - t2 (s)" class="DigNum (strict)"(error in=w209, "Value"=w200) -> (error out=w210:errorcluster)  [unwired: 1 in, 1 out]
            n85 = property on="Input \nVoltage 2 \n- Vin2 (V)" class="DigNum (strict)"(error in=w226, "Value"=w224) -> (error out=w227:errorcluster)  [unwired: 1 in, 1 out]
            n86 = property on="Duration of the pulse (s)" class="DigNum (strict)"(error in=w210, "Value"=w201) -> (error out=w211:errorcluster)  [unwired: 1 in, 1 out]
            n87 = property on="Input Voltage (V)" class="DigNum (strict)"(error in=w227, "Value"=w223) -> (error out=w228:errorcluster)  [unwired: 1 in, 1 out]
            n88 = property on="Save Scope Raw Data?" class="Bool (strict)"(error in=w211, "Value"=w207) -> (error out=w208:errorcluster)  [unwired: 1 in, 1 out]
            n89 = property on="Nominal Output Voltage (V)" class="DigNum (strict)"(error in=w228, "Value"=w222) -> (error out=w229:errorcluster)  [unwired: 1 in, 1 out]
            n90 = property on="Auto Scale Y-Axis?" class="Bool (strict)"(error in=w208, "Value"=w206) -> (error out=w203:errorcluster)  [unwired: 1 in, 1 out]
            n91 = property on="Voltage to \nsettle above Vnom (V)" class="DigNum (strict)"(error in=w229, "Value"=w221) -> (error out=w230:errorcluster)  [unwired: 1 in, 1 out]
            n92 = property on="Shunt Resistance (Ohm)" class="DigNum (strict)"(error in=w203, "Value"=w204) -> (error out=w205:errorcluster)  [unwired: 1 in, 1 out]
            n93 = Compound Arithmetic op=ADD(w199, w200, w201) -> (w198:dbl)
            n94 = property on="Percentage \nof Vnom (%)" class="DigNum (strict)"(error in=w230, "Value"=w220) -> (error out=w234:errorcluster)  [unwired: 1 in, 1 out]
            n95 = Multiply(x=w198, y=5.0) -> (x*y=w196:dbl)
            n96 = Type Cast(type=enum32{"Item 0", "Item 1"}."Item 0" ("Settling Time Calculation"), x=w219) -> (*(type *) &x=w217:enum32{"Item 0", "Item 1"})
            n97 = Bundle By Name(cluster=w231, "Test Inputs.Advance Setting"=w233) -> (w232:T17)
            n98 = property on="Sequence Timeout" class="DigNum (strict)"(error in=w205, "Value"=w196) -> (error out=w202:errorcluster)  [unwired: 1 in, 1 out]
            n99 = property on="Settling Time Calculation" class="RadioBtnsControl (strict)"(error in=w234, "Value"=w217) -> (error out=w214:errorcluster)  [unwired: 1 in, 1 out]
            n100 = property on="Take Transient snapshot?" class="Bool (strict)"(error in=w214, "Value"=w215) -> (error out=w216:errorcluster)  [unwired: 1 in, 1 out]
            n101 = Merge Errors(w216, w202) -> (w213:errorcluster)
          }
          event "Tab Enum": Value Change {
            n102 = event-data() -> ("NewVal"=→"Tab Control":T1)  [unwired: 1 in]
          }
          event "Advanced Settings": Value Change {
            n103 = event-data() -> ()  [unwired: 1 in, 1 out]
            n104 = Unbundle By Name(w241) -> ("Test Inputs.Advance Setting"=w243:T12)
            n105 = call "Advance Settings UI.vi"("Advance Setting In"=w243, "error in (no error)"=w244) -> ("Advance Setting Out"=w238:T12, "error out"=w240:errorcluster)  [unwired: 12 in]
            n106 = Bundle By Name(cluster=w241, "Test Inputs.Advance Setting"=w238) -> (w242:T17)
            n107 = property on="Advance Setting" class="Clust (strict)"(error in=w240, "Value"=w238) -> (error out=w239:errorcluster)  [unwired: 1 in, 1 out]
          }
          event "Shunt Resistance (Ohm)": Value Change {
            n108 = event-data() -> ("NewVal"=w245:dbl)  [unwired: 1 in]
            n109 = property on="Shunt Resistance (Ohm)" class="DigNum (strict)"(error in=w247, "Value"=w245) -> (error out=w246:errorcluster)  [unwired: 1 in, 1 out]
          }
        }
      }
      frame "----------------- Macro ---------------" {
        # "Not used. category splitter"
      }
      frame "Macro: Initialize" {
        w257 = string[] ["Macro: GUI Start"]  # Standalone: Start the debug
        w258 = string[] ["Macro: Execute Test", "Exit"]  # Automation: Execute and stop
        # "Hidden in UI"
        # "This case decides the mode of the execution. Debug Mode: The plugin will act as a standalone GUI where user can change inputs, run test and debug the system. automation mode: The plugin will act as a flat code and go through all the test procedures and stops."
        n110 = call <userlib>:"Get Mode.vi"("Caller Information"="Caller Information", "error in (no error)"=w260) -> ("Automation(F) \\ Standalone (T)"=w256:bool, "error out"=w259:errorcluster)  [unwired: 12 in]
        n111 = Bundle By Name(cluster=w264, "Termination Monitor Info.Caller Information"="Caller Information") -> (w253:T17)
        n112 = Select(t=w257, s=w256, f=w258) -> (s? t:f=w255:string[])
        n113 = call <userlib>:"Enqueue.vi"("Queue in"=w262, "States"=w255, "Enqueue at Front?(F)"=TRUE, "error in (no error)"=w259) -> ("error out"=w263:errorcluster)  [unwired: 10 in, 1 out]
      }
      frame "Macro: Execute Test" {
        w265 = string[] ["TerminationMonitor: Start", "Test: Start", "Test: Get Current Measurement Option", "Test: Prepare Source SMU", "Test: Prepare Load SMU", "Test: Prepare Scope", "Test: Create Load Current Seq", "Test: Check Sequence Size", "Test: Check Buffer and on-board Size", "Test: Set Input Voltage", "Test: Calc Min Delay for Max. Ref Position", "Test: Generate Load Current Sequence", "Test: Measure Transient", "Test: Calculate Out. Voltage Threshold", "Test: Calculate Settling Time", "Test: Cleanup DCPower", "Test: Cleanup Scope", "Test: Update UI", "Test: End", "TerminationMonitor: Stop"]  # Test Procedure
        # "List the states required for the test procedure. This state will be called in both automation mode and standalone mode when requested to run the test.\nDont remove 'Test: Start' and 'Test: End'."
        n114 = call <userlib>:"Enqueue.vi"("Queue in"=w274, "States"=w265, "Enqueue at Front?(F)"=TRUE, "error in (no error)"=w275) -> ("error out"=w267:errorcluster)  [unwired: 10 in, 1 out]
        n115 = Array Size(array=w265) -> (size(s)=w269:i32)
        n116 = call "Progress Monitor.vi"("State Array []"=w265, "Option (Default: Get State Index)"=Progress_Monitor_Option."State Array Init" ("Option")) -> ()  [unwired: 13 in, 1 out]
        n117 = property on="Progress" class="Slide (strict)"(error in=w267, "Visible"=TRUE, "Scale.Maximum"=w269, "Value"=0 ("Progress")) -> (error out=w266:errorcluster)  [unwired: 1 in, 1 out]
      }
      frame "Macro: GUI Start" {
        # "Initialize the data cluster for the standalone mode and register for the event from caller.\nDon't remove 'GUI: Initialize Data' and 'GUI: Register Event'."
        n118 = call <userlib>:"Enqueue.vi"("Queue in"=w279, "States"=string[] ["GUI: Initialize Data", "GUI: Register Event"], "Enqueue at Front?(F)"=TRUE, "error in (no error)"=w281) -> ("error out"=w282:errorcluster)  [unwired: 10 in, 1 out]
      }
      frame "Macro: GUI Stop" {
        # "Cleanups the standalone mode and stop the execution.\nDon't remove 'GUI: Unregister Event', 'GUI: Cleanup Data' and 'Exit'."
        n119 = call <userlib>:"Enqueue.vi"("Queue in"=w286, "States"=string[] ["GUI: Unregister Event", "GUI: Cleanup Data", "Exit"], "Enqueue at Front?(F)"=TRUE, "error in (no error)"=w288) -> ("error out"=w289:errorcluster)  [unwired: 10 in, 1 out]
      }
      frame "--------------- GUI Mode-----------------" {
        # "Not used. category splitter"
      }
      frame "GUI: Initialize Data" {
        w317 = dbl[] []  # Load Current Waveform
        w319 = T1."Station Setup" ("Tab Enum")
        w322 = string[][] []  # Test Results[][]
        w332 = T14 {"Measured Output Voltage"={"x-axis"=[], "wfm"=[]}, "Measured Load Current"={"x-axis"=[], "wfm"=[]}, "Actual Sample Rate in S/s"=0.0, "First Edge - Settling Time in s"=0.0, "Second Edge - Settling Time in s"=0.0}  # Test Results
        # "Add the front panel controls terminal here and connect them to the bundle structure, So they will be available through data cluster in every case. If the controls and indicators are added to the 'Test Inputs' & 'Test Results' cluster then they are already available in the data cluster since they are typedefs."
        n120 = property on="Run" class="Bool (strict)"(error in=w326, "DisabledEnum"=T19."Enabled" ("Disabled")) -> (error out=w329:errorcluster)  [unwired: 1 in, 1 out]
        n121 = local write "Tab Enum"(w319) -> ()
        n122 = local write "Tab Control"(w319) -> ()
        n123 = property on="Terminate" class="Bool (strict)"(error in=w329, "DisabledEnum"=T19."Disabled and Grayed Out" ("Disabled")) -> (error out=w325:errorcluster)  [unwired: 1 in, 1 out]
        n124 = property on="Progress" class="Slide (strict)"(error in=w325, "Visible"=FALSE) -> (error out=w324:errorcluster)  [unwired: 1 in, 1 out]
        n125 = Bundle By Name(cluster=w331, "Test Pins"="Test Pins", "Test Inputs"="Test Inputs", "Test Results"=w332, "Test Results[][]"=w322, "Logger Folder Path"="DataLogPath", "Load Current Waveform"=w317) -> (w316:T17)
        n126 = control-ref of="Settling Time Calculation"() -> (w301:refnum<vi>)
        n127 = control-ref of="Auto Scale Y-Axis?"() -> (w300:refnum<vi>)
        n128 = control-ref of="Save Scope Raw Data?"() -> (w299:refnum<vi>)
        n129 = control-ref of="Take Transient snapshot?"() -> (w298:refnum<vi>)
        n130 = control-ref of="Advanced Settings"() -> (w297:refnum<vi>)
        n131 = control-ref of="SystemSetup"() -> (w314:refnum<vi>)
        n132 = control-ref of="Sequence Timeout"() -> (w296:refnum<vi>)
        n133 = control-ref of="First Edge - Settling Time (s)"() -> (w295:refnum<vi>)
        n134 = control-ref of="Second Edge - Settling Time (s)"() -> (w294:refnum<vi>)
        n135 = control-ref of="Shunt Resistance (Ohm)"() -> (w312:refnum<vi>)
        n136 = control-ref of="Input Voltage (V)"() -> (w310:refnum<vi>)
        n137 = control-ref of="Load Current 1 - Iload1 (A)"() -> (w309:refnum<vi>)
        n138 = control-ref of="Load Current 2 - Iload2 (A)"() -> (w308:refnum<vi>)
        n139 = control-ref of="Delay - t1 (s)"() -> (w307:refnum<vi>)
        n140 = control-ref of="Duration of the pulse (s)"() -> (w306:refnum<vi>)
        n141 = control-ref of="Delay - t2 (s)"() -> (w305:refnum<vi>)
        n142 = control-ref of="Nominal Output Voltage (V)"() -> (w304:refnum<vi>)
        n143 = control-ref of="Voltage to settle above Vnom (V)"() -> (w303:refnum<vi>)
        n144 = control-ref of="Percentage of Vnom (%)"() -> (w302:refnum<vi>)
        n145 = control-ref of="Shunt Resistance Info"() -> (w311:refnum<vi>)
        n146 = Build Array(w314, w312, w311, w310, w309, w308, w307, w306, w305, w304, w303, w302, w301, w300, w299, w298, w297, w296, w295, w294) -> (w313:refnum<vi>[])
        n147 = Bundle By Name(cluster=w316, "UI Ctls"=w313) -> (w315:T17)
      }
      frame "GUI: Register Event" {
        # "Hidden in UI"
        # "Register for the events from caller."
        n148 = register-events(error in=w337, "Caller Events") -> (reference out=w334:refnum<event-registration>, error out=w335:errorcluster)  [unwired: 1 in]
      }
      frame "GUI: Unregister Event" {
        n149 = Unregister For Events(event registration refnum=w338, error in=w341) -> (error out=w339:errorcluster)
      }
      frame "GUI: Cleanup Data" {
        # "Cleanup the reference or other resources before exiting"
      }
      frame "GUI: Set Busy" {
        n150 = call "Progress Monitor.vi"("State"=w345) -> ("State Array Index"=w348:i32)  [unwired: 14 in]
        n151 = property on="Progress" class="Slide (strict)"(error in=w346, "Value"=w348) -> (error out=w347:errorcluster)  [unwired: 1 in, 1 out]
        n152 = Unbundle By Name(w349) -> ("UI Ctls"=w354:refnum<vi>[])
        n153 = for {
          tunnel: [w359] -> w355 mode=indexing
          tunnel: w347 -> [w360]
          tunnel: w354 -> [w358] mode=indexing
          tunnel: T19."Disabled and Grayed Out" ("Disabled") -> [w357]
          n154 = property class="Ctl"(reference=w358, error in=w360, "DisabledEnum"=w357) -> (error out=w359:errorcluster)  [unwired: 1 out]
        }
        n155 = Merge Errors(w355) -> (w352:errorcluster)
        n156 = call "Defer Front Panel.vi"("Defer Front Panel?"=TRUE, "error in"=w352) -> ("error out"=w350:errorcluster)  [unwired: 13 in]
      }
      frame "GUI: Unset Busy" {
        n157 = call "Progress Monitor.vi"("State"=w361) -> ("State Array Index"=w362:i32)  [unwired: 14 in]
        n158 = property on="Progress" class="Slide (strict)"(error in=w363, "Value"=w362) -> (error out=w364:errorcluster)  [unwired: 1 in, 1 out]
        n159 = Unbundle By Name(w365) -> ("UI Ctls"=w370:refnum<vi>[])
        n160 = for {
          tunnel: [w375] -> w371 mode=indexing
          tunnel: w364 -> [w376]
          tunnel: w370 -> [w374] mode=indexing
          tunnel: T19."Enabled" ("Disabled") -> [w373]
          n161 = property class="Ctl"(reference=w374, error in=w376, "DisabledEnum"=w373) -> (error out=w375:errorcluster)  [unwired: 1 out]
        }
        n162 = Merge Errors(w371) -> (w367:errorcluster)
        n163 = call "Defer Front Panel.vi"("Defer Front Panel?"=FALSE, "error in"=w367) -> ("error out"=w366:errorcluster)  [unwired: 13 in]
      }
      frame "GUI: Update Shunt Resistance Display" {
        n164 = Unbundle By Name(w380) -> ("Current Measurement Option"=w377:T16)
        n165 = case shown="\"Scope Measurement\"" w377 {
          tunnel: w378 -> [w385 w389]
          tunnel: [w383 w387] -> w379
          frame "SMU Measurement" {
            w382 = FALSE ("Visible")
            n166 = property on="Shunt Resistance (Ohm)" class="DigNum (strict)"(error in=w385, "Visible"=w382) -> (error out=w384:errorcluster)  [unwired: 1 in, 1 out]
            n167 = property on="Shunt Resistance Info" class="Ring (strict)"(error in=w384, "Visible"=w382) -> (error out=w383:errorcluster)  [unwired: 1 in, 1 out]
          }
          frame "Scope Measurement" {
            w386 = TRUE ("Visible")
            # "Adding info since tip will not be displayed in IS"
            n168 = property on="Shunt Resistance (Ohm)" class="DigNum (strict)"(error in=w389, "Visible"=w386) -> (error out=w388:errorcluster)  [unwired: 1 in, 1 out]
            n169 = property on="Shunt Resistance Info" class="Ring (strict)"(error in=w388, "Visible"=w386) -> (error out=w387:errorcluster)  [unwired: 1 in, 1 out]
          }
        }
      }
      frame "GUI: Update Sequence Timeout" {
        # "Multiply by 5 to have sufficient timeout"
        n170 = Unbundle By Name(w398) -> ("Test Inputs.Delay - t1 in s"=w397:dbl, "Test Inputs.Delay - t2 in s"=w396:dbl, "Test Inputs.Duration of the pulse in Second"=w395:dbl)
        n171 = Compound Arithmetic op=ADD(w397, w396, w395) -> (w390:dbl)
        n172 = Multiply(x=w390, y=5.0) -> (x*y=w394:dbl)
        n173 = property on="Sequence Timeout" class="DigNum (strict)"(error in=w391, "Value"=w394) -> (error out=w392:errorcluster)  [unwired: 1 in, 1 out]
      }
      frame "GUI: Get Logger File Path" {
        n174 = Unbundle By Name(w400) -> ("Logger Folder Path"=w407:path)
        n175 = call <vilib>:"Check if File or Folder Exists.vi"("error in (no error)"=w403, "path"=w407) -> ("error out"=w406:errorcluster, "file or folder exists?"=w405:bool, "dup path"=w404:path)  [unwired: 7 in]
        n176 = case shown="True" w405 {
          tunnel: [w410 w419] -> w402
          tunnel: w406 -> [w410 w422]
          tunnel: w400 -> [w409 w426]
          tunnel: [w409 w425] -> w401
          tunnel: w404 -> [_ w421]
          frame False {
          }
          frame True {
            n177 = Strip Path(path=w421) -> (name=w413:string)  [unwired: 1 out]
            n178 = call "Get Unique Name.vi"() -> ("date"=w420:string, "Unique String"=w412:string)  [unwired: 14 in]
            n179 = Concatenate Strings(w413, w420) -> (w416:string)
            n180 = Concatenate Strings(w413, w412) -> (w411:string)
            n181 = Concatenate Strings(w416, "\\" ("string"), w411) -> (w423:string)
            n182 = Build Path(base path=w421, name or relative path=w423) -> (appended path=w418:path)
            n183 = call <vilib>:"Create Directory Recursive.vi"("error in (no error)"=w422, "directory"=w418) -> ("error out"=w419:errorcluster, "directory copy"=w415:path)  [unwired: 3 in, 1 out]
            n184 = Build Path(base path=w415, name or relative path=w411) -> (appended path=w414:path)
            n185 = Bundle By Name(cluster=w426, "Valid Logger Path?"=TRUE ("Valid Logger path?"), "Logger File Path"=w414) -> (w425:T17)
          }
        }
      }
      frame "GUI: Log" {
        n186 = Unbundle By Name(w434) -> ("Test Inputs.Save Scope Raw Data?"=w427:bool, "Valid Logger Path?"=w428:bool, "Test Inputs"=w430:T10, "Test Results"=w431:T14, "Logger File Path"=w429:path)
        n187 = case shown="True" w428 {
          tunnel: [w436 w442] -> w433
          tunnel: w432 -> [w436 w441]
          tunnel: w431 -> [_ w440]
          tunnel: w430 -> [_ w439]
          tunnel: w429 -> [_ w438]
          tunnel: w427 -> [_ w437]
          frame False {
          }
          frame True {
            n188 = call "Log Data.vi"("Test Inputs"=w439, "Save Scope Raw Data?"=w437, "Test Results"=w440, "DataLogger File Path"=w438, "error in (no error)"=w441) -> ("error out"=w442:errorcluster)  [unwired: 10 in]
          }
        }
      }
      frame "GUI: Update Graph Scale" {
        w456 = u32 1 ("Active Plot")
        w457 = u32 0 ("Active Plot")
        # "Placing plot legend inside graph in top right"
        n189 = Unbundle By Name(w459) -> ("Test Inputs.Auto Scale Y-Axis?"=w458:bool)
        n190 = control-ref of="Load Transient"() -> (w444:refnum<vi>)
        n191 = property class="XYGraph (strict)"(reference=w444, error in=w445) -> (reference out=w453:refnum<vi>, error out=w454:errorcluster, "Left"=w452:i32, "Top"=w451:i32)
        n192 = Add(x=w451, y=11) -> (x+y=w447:i32)
        n193 = Add(x=w452, y=418) -> (x+y=w448:i32)
        n194 = property on="Property Node" class="XYGraph (strict)"(reference=w453, error in=w454, "Active Plot"=w457, "Plot.YScaleIdx"=w457, "Active Plot"=w456, "Plot.YScaleIdx"=w456, "LegLeft"=w448, "LegTop"=w447) -> (reference out=w446:refnum<vi>, error out=w455:errorcluster)
        n195 = case shown="True" w458 {
          tunnel: [w461 w464] -> w443
          tunnel: w455 -> [w461 w463]
          tunnel: w446 -> [_ w462]
          frame False {
          }
          frame True {
            n196 = call "Two Plot XY Graph Auto Scale.vi"("Two Plot XY Graph Ref In"=w462, "error in (no error)"=w463) -> ("error out"=w464:errorcluster)  [unwired: 12 in, 1 out]
          }
        }
      }
      frame "GUI: Log Waveform Snapshot" {
        n197 = Unbundle By Name(w465) -> ("Test Inputs.Save Transient Graph?"=w471:bool, "Valid Logger Path?"=w469:bool, "Logger File Path"=w468:path)
        n198 = And(x=w471, y=w469) -> (x .and. y?=w470:bool)
        n199 = case shown="True" w470 {
          tunnel: w466 -> [w473 w475]
          tunnel: [w473 w474] -> w467
          tunnel: w468 -> [_ w476]
          frame False {
          }
          frame True {
            w482 = T21 {"Major Color"=14737632, "Minor Color"=15987699} ("Y Scale.Grid Colors")
            w483 = T21 {"Major Color"=16777216, "Minor Color"=16777216} ("Y Scale.Grid Colors")
            n200 = control-ref of="Load Transient"() -> (w477:refnum<vi>)
            n201 = Path To String(path=w476) -> (string=w494:string)
            n202 = property class="XYGraph (strict)"(reference=w477, error in=w475, "ActYScl"=0 ("Active Y Scale"), "YScale.GridColors"=w483, "ActYScl"=1 ("Active Y Scale"), "YScale.GridColors"=w483) -> (reference out=w486:refnum<vi>, error out=w487:errorcluster)
            n203 = Concatenate Strings(w494, "_Waveform" ("string"), ".bmp" ("format string")) -> (w495:string)
            n204 = String To Path(string=w495) -> (path=w493:path)
            n205 = invoke class="XYGraph (strict)" method="Export Image"(reference=w486, error in=w487, "FileType"=enum32{"BMP", "EPS", "EMF", "PICT"}."BMP" ("File Type"), "Target"=enum32{"File", "Clipboard"}."File", "Path"=w493, "HideGrid"=TRUE ("Hide Grid")) -> (reference out=w478:refnum<vi>, error out=w479:errorcluster)  [unwired: 2 in, 6 out]
            n206 = property class="XYGraph (strict)"(reference=w478, error in=w479, "ActYScl"=0 ("Active Y Scale"), "YScale.GridColors"=w482, "ActYScl"=1 ("Active Y Scale"), "YScale.GridColors"=w482) -> (error out=w474:errorcluster)  [unwired: 1 out]
          }
        }
      }
      frame "GUI: Start Test" {
        n207 = property on="Run" class="Bool (strict)"(error in=w498, "DisabledEnum"=T19."Disabled and Grayed Out" ("Disabled")) -> (error out=w503:errorcluster)  [unwired: 1 in, 1 out]
        n208 = property on="Terminate" class="Bool (strict)"(error in=w503, "DisabledEnum"=T19."Enabled" ("Disabled")) -> (error out=w501:errorcluster)  [unwired: 1 in, 1 out]
        n209 = property on="Progress" class="Slide (strict)"(error in=w501, "Visible"=TRUE, "Value"=0 ("Progress")) -> (error out=w499:errorcluster)  [unwired: 1 in, 1 out]
      }
      frame "GUI: End Test" {
        n210 = property on="Run" class="Bool (strict)"(error in=w507, "Value"=FALSE ("Run"), "DisabledEnum"=T19."Enabled" ("Disabled")) -> (error out=w513:errorcluster)  [unwired: 1 in, 1 out]
        n211 = property on="Terminate" class="Bool (strict)"(error in=w513, "DisabledEnum"=T19."Disabled and Grayed Out" ("Disabled")) -> (error out=w512:errorcluster)  [unwired: 1 in, 1 out]
        n212 = property on="Progress" class="Slide (strict)"(error in=w512, "Visible"=FALSE) -> (error out=w506:errorcluster)  [unwired: 1 in, 1 out]
      }
      frame "------------ TerminationMonitor -----------" {
        # "Not used. category splitter"
      }
      frame "TerminationMonitor: Start" {
        # "Termination Monitor monitors the execution of the caller. Use Termination Monitor Status to get the termination status. If the caller is terminating, stop the test procedure, cleanup and stop."
        n213 = Unbundle By Name(w521) -> ("Termination Monitor Info.Caller Information"=w520:T7)
        n214 = call <userlib>:"Termination Monitor Start.vi"("Caller Information"=w520, "error in (no error)"=w523) -> ("Termination Monitor Info out"=w519:T15, "error out"=w524:errorcluster)  [unwired: 12 in]
        n215 = Bundle By Name(cluster=w521, "Termination Monitor Info"=w519) -> (w522:T17)
      }
      frame "TerminationMonitor: Stop" {
        n216 = Unbundle By Name(w528) -> ("Termination Monitor Info"=w527:T15)
        n217 = call <userlib>:"Termination Monitor Stop.vi"("Status Info in"=w527, "error in (no error)"=w530) -> ("Status Info out"=w526:T15, "error out"=w531:errorcluster)  [unwired: 12 in]
        n218 = Bundle By Name(cluster=w528, "Termination Monitor Info"=w526) -> (w529:T17)
      }
      frame "------------ Automation Mode -----------" {
        # "Not used. category splitter"
      }
      frame "Test: Start" {
        # "Reinitialize/Reset/Update the data from the UI to the data cluster so that the data will be considered for the test procedure.\nReset the Test Results."
        n219 = call "Progress Monitor.vi"("State"=w537) -> ("State Array Index"=w540:i32)  [unwired: 14 in]
        n220 = property on="Progress" class="Slide (strict)"(error in=w538, "Value"=w540) -> (error out=w539:errorcluster)  [unwired: 1 in, 1 out]
        n221 = local read "DataLogPath"() -> (w541:path)
        n222 = local read "Test Inputs"() -> (w552:T10)
        n223 = local read "Test Pins"() -> (w542:T6)
        n224 = property on="Run" class="Bool (strict)"(error in=w539, "DisabledEnum"=T19."Disabled and Grayed Out" ("Disabled")) -> (error out=w548:errorcluster)  [unwired: 1 in, 1 out]
        n225 = Bundle By Name(cluster=w553, "Test Pins"=w542, "Test Inputs"=w552, "Test Results"=T14 {"Measured Output Voltage"={"x-axis"=[], "wfm"=[]}, "Measured Load Current"={"x-axis"=[], "wfm"=[]}, "Actual Sample Rate in S/s"=0.0, "First Edge - Settling Time in s"=0.0, "Second Edge - Settling Time in s"=0.0}, "Logger Folder Path"=w541, "Sequence name"="CurrentSequence") -> (w543:T17)
        n226 = property on="Terminate" class="Bool (strict)"(error in=w548, "DisabledEnum"=T19."Enabled" ("Disabled")) -> (error out=w545:errorcluster)  [unwired: 1 in, 1 out]
        n227 = property on="Progress" class="Slide (strict)"(error in=w545, "Visible"=FALSE) -> (error out=w544:errorcluster)  [unwired: 1 in, 1 out]
      }
      frame "Test: Get Current Measurement Option" {
        # "Get Measurement option based on Pin selected"
        n228 = call "Progress Monitor.vi"("State"=w554) -> ("State Array Index"=w557:i32)  [unwired: 14 in]
        n229 = property on="Progress" class="Slide (strict)"(error in=w555, "Value"=w557) -> (error out=w556:errorcluster)  [unwired: 1 in, 1 out]
        n230 = Unbundle By Name(w559) -> ("Test Pins.Measure Load Current"=w562:string)
        n231 = call "Get Current Measurement Option.vi"("Capture Load Current Waveform"=w562, "error in (no error)"=w556) -> ("Current Measurement Option"=w558:T16, "error out"=w561:errorcluster)  [unwired: 12 in]
        n232 = Bundle By Name(cluster=w559, "Current Measurement Option"=w558) -> (w560:T17)
      }
      frame "Test: Prepare Source SMU" {
        n233 = call "Progress Monitor.vi"("State"=w567) -> ("State Array Index"=w570:i32)  [unwired: 14 in]
        n234 = property on="Progress" class="Slide (strict)"(error in=w568, "Value"=w570) -> (error out=w569:errorcluster)  [unwired: 1 in, 1 out]
        n235 = Unbundle By Name(w571) -> ("Test Pins.Set Input Voltage"=w564:string, "Test Inputs.Input Voltage in V"=w565:dbl)
        n236 = call "Prepare Source.vi"("Set Vin"=w564, "Initial Voltage Level (V)"=w565, "error in (no error)"=w569) -> ("error out"=w566:errorcluster)  [unwired: 12 in]
      }
      frame "Test: Prepare Load SMU" {
        w574 = 1025 items=["Automatically after Source Complete"=1025, "On Demand"=1026, "On Measure Trigger"=1027] ("Measurement:Advanced:Measure When")
        w587 = T22 1030 items=["Source Complete Event"=1030, "Measure Complete Event"=1031, "Sequence Iteration Complete Event"=1032, "Sequence Engine Done Event"=1033, "Pulse Complete Event"=1051, "Ready For Pulse Trigger Event"=1052] ("event")
        w594 = TRUE  # output enabled
        w599 = T23 1006 items=["DC Voltage"=1006, "DC Current"=1007, "Pulse Voltage"=1049, "Pulse Current"=1050] ("output function")
        w596 = T24 1020 items=["Single Point"=1020, "Sequence"=1021] ("source mode")
        # "By default measurement is acquired On Demand\nTo configure Record Length set Automatically after source complete"
        # "Set Voltage 0 to\nsink SMU"
        n237 = call "Progress Monitor.vi"("State"=w602) -> ("State Array Index"=w605:i32)  [unwired: 14 in]
        n238 = Unbundle By Name(w608) -> ("Test Inputs.Advance Setting.Prepare.Load SMU Record Length"=w573:i32, "Test Inputs.Load Current 1 in A"=w606:dbl, "Test Pins.Set Load Current"=w607:string)
        n239 = property on="Progress" class="Slide (strict)"(error in=w603, "Value"=w605) -> (error out=w604:errorcluster)  [unwired: 1 in, 1 out]
        n240 = call "Pin Name to Reference.vim"("Pin Name"=w607, "type"=refnum<k15> refnum ("instrument handle"), "error in (no error)"=w604) -> ("Reference"=w588:refnum<k15>, "error out"=w589:errorcluster)  [unwired: 7 in, 4 out]
        n241 = Absolute Value(x=w606) -> (abs(x)=w583:dbl)
        n242 = call <instrlib>:"niDCPower Abort With Channels.vi"("error in (no error)"=w589, "instrument handle"=w588) -> ("error out"=w600:errorcluster, "instrument handle out"=w601:refnum<k15>)  [unwired: 8 in]
        n243 = call <instrlib>:"niDCPower Configure Source Mode With Channels.vi"("error in (no error)"=w600, "source mode"=w596, "instrument handle"=w601) -> ("error out"=w598:errorcluster, "instrument handle out"=w597:refnum<k15>)  [unwired: 7 in]
        n244 = call <instrlib>:"niDCPower Configure Output Function.vi"("error in (no error)"=w598, "output function"=w599, "instrument handle"=w597) -> ("error out"=w595:errorcluster, "instrument handle out"=w581:refnum<k15>)  [unwired: 7 in]
        n245 = call <instrlib>:"niDCPower Configure Voltage Level.vi"("error in (no error)"=w595, "voltage level"=0.0 ("voltage limit"), "instrument handle"=w581) -> ("error out"=w582:errorcluster, "instrument handle out"=w580:refnum<k15>)  [unwired: 7 in]
        n246 = call <instrlib>:"niDCPower Configure Current Limit.vi"("error in (no error)"=w582, "current limit"=w583, "instrument handle"=w580) -> ("error out"=w593:errorcluster, "instrument handle out"=w591:refnum<k15>)  [unwired: 7 in]
        n247 = call <instrlib>:"niDCPower Configure Output Enabled.vi"("error in (no error)"=w593, "output enabled"=w594, "instrument handle"=w591) -> ("error out"=w592:errorcluster, "instrument handle out"=w577:refnum<k15>)  [unwired: 7 in]
        n248 = property class="niDCPower"(reference=w577, error in=w592, "Sequence Loop Count"=1 ("Source:Advanced:Sequence Loop Count"), "Measure When"=w574, "Measure Record Length"=w573) -> (reference out=w576:refnum<k15>, error out=w578:errorcluster)
        n249 = call <instrlib>:"niDCPower Initiate.vi"("error in (no error)"=w578, "instrument handle"=w576) -> ("error out"=w586:errorcluster, "instrument handle out"=w585:refnum<k15>)  [unwired: 8 in]
        n250 = call <instrlib>:"niDCPower Wait For Event With Channels.vi"("error in (no error)"=w586, "event"=w587, "instrument handle"=w585) -> ("error out"=w584:errorcluster)  [unwired: 7 in, 1 out]
      }
      frame "Test: Prepare Scope" {
        # "Set sampling rate"
        # "Aborting prev acquisition"
        n251 = Unbundle By Name(w628) -> ("Current Measurement Option"=w618:T16, "Test Pins.Measure Load Current"=w619:string, "Test Pins.Measure Output Voltage"=w635:string)
        n252 = call "Progress Monitor.vi"("State"=w630) -> ("State Array Index"=w633:i32)  [unwired: 14 in]
        n253 = property on="Progress" class="Slide (strict)"(error in=w631, "Value"=w633) -> (error out=w632:errorcluster)  [unwired: 1 in, 1 out]
        n254 = call "Pin Name to Reference.vim"("Pin Name"=w635, "type"=refnum<k15> refnum ("instrument handle"), "error in (no error)"=w632) -> ("Reference"=w615:refnum<k15>, "Channel"=w612:string, "error out"=w626:errorcluster)  [unwired: 7 in, 3 out]
        n255 = call <instrlib>:"niScope Abort.vi"("instrument handle"=w615, "error in"=w626) -> ("instrument handle out"=w614:refnum<k15>, "error out"=w616:errorcluster)  [unwired: 12 in]
        n256 = property class="niScope"(reference=w614, error in=w616, "Active Channel"=w612, "Channel Enabled"=TRUE ("Vertical:Channel Enabled")) -> (reference out=w617:refnum<k15>, error out=w622:errorcluster, "Vertical Coupling"=w610:i32)
        n257 = case shown="\"SMU Measurement\"" w618 {
          tunnel: w622 -> [w646 w653]
          tunnel: [w645 w653] -> w621
          tunnel: [w644 w652] -> w620
          tunnel: w619 -> [w643 _]
          tunnel: w617 -> [_ w652]
          tunnel: [w639 w651] -> w613
          tunnel: w612 -> [w637 w651]
          frame "Scope Measurement" {
            n258 = call "Pin Name to Reference.vim"("Pin Name"=w643, "type"=refnum<k15> refnum ("instrument handle"), "error in (no error)"=w646) -> ("Reference"=w648:refnum<k15>, "Channel"=w638:string, "error out"=w649:errorcluster)  [unwired: 7 in, 3 out]
            n259 = Build Array(w637, w638) -> (w640:string[])
            n260 = property class="niScope"(reference=w648, error in=w649, "Active Channel"=w638, "Channel Enabled"=TRUE ("Vertical:Channel Enabled")) -> (reference out=w644:refnum<k15>, error out=w645:errorcluster)
            n261 = Array To Spreadsheet String(delimiter (Tab)=",", array=w640, 3:"" ("format string")) -> (spreadsheet string=w639:string)
          }
          frame "SMU Measurement" {
          }
        }
        n262 = property class="niScope"(reference=w620, error in=w621) -> (reference out=w623:refnum<k15>, error out=w624:errorcluster, "Actual Sample Rate"=w611:dbl)
        n263 = property class="niScope"(reference=w623, error in=w624, "Min Sample Rate"=w611) -> (error out=w634:errorcluster)  [unwired: 1 out]
        n264 = Bundle By Name(cluster=w628, "Scope Channels"=w613, "Output Voltage Coupling"=w610) -> (w629:T17)
      }
      frame "Test: Create Load Current Seq" {
        # "Duration of each step is  [Source Delay + (Aperture Time * Record Length)]\nNo. of steps is calculated by  Duration of each pulse/ [Source Delay + (Aperture Time * Record Length)]"
        n265 = Unbundle By Name(w680) -> ("Test Inputs.Load Current 1 in A"=w687:dbl, "Test Inputs.Load Current 2 in A"=w686:dbl, "Test Inputs.Delay - t1 in s"=w679:dbl, "Test Inputs.Duration of the pulse in Second"=w685:dbl, "Test Inputs.Delay - t2 in s"=w656:dbl, "Test Pins.Set Load Current"=w684:string)
        n266 = call "Progress Monitor.vi"("State"=w675) -> ("State Array Index"=w678:i32)  [unwired: 14 in]
        n267 = property on="Progress" class="Slide (strict)"(error in=w676, "Value"=w678) -> (error out=w677:errorcluster)  [unwired: 1 in, 1 out]
        n268 = call "Pin Name to Reference.vim"("Pin Name"=w684, "type"=refnum<k15> refnum ("instrument handle"), "error in (no error)"=w677) -> ("Reference"=w667:refnum<k15>, "Channel"=w665:string, "error out"=w668:errorcluster)  [unwired: 7 in, 3 out]
        n269 = property class="niDCPower"(reference=w667, error in=w668, "Active Channel"=w665) -> (error out=w683:errorcluster, "Source Delay"=w666:dbl, "Aperture Time"=w657:dbl, "Measure Record Length"=w664:i32)  [unwired: 1 out]
        n270 = To Double Precision Float(number=w664) -> (double precision float=w663:dbl)
        n271 = Multiply(x=w657, y=w663) -> (x*y=w655:dbl)
        n272 = Add(x=w666, y=w655) -> (x+y=w654:dbl)
        n273 = Divide(x=w679, y=w654) -> (x/y=w662:dbl)
        n274 = Divide(x=w685, y=w654) -> (x/y=w660:dbl)
        n275 = Divide(x=w656, y=w654) -> (x/y=w659:dbl)
        n276 = To Long Integer(number=w660) -> (32bit integer=w673:i32)
        n277 = To Long Integer(number=w659) -> (32bit integer=w661:i32)
        n278 = To Long Integer(number=w662) -> (32bit integer=w672:i32)
        n279 = Initialize Array(w686, w673) -> (w671:dbl[])
        n280 = Initialize Array(w687, w661) -> (w658:dbl[])
        n281 = Build Array(w679, w685, w656) -> (w674:dbl[])
        n282 = Initialize Array(w687, w672) -> (w670:dbl[])
        n283 = Build Array (concatenate)(w670, w671, w658) -> (w682:dbl[])
        n284 = Bundle By Name(cluster=w680, "Load Current Waveform"=w682, "Load Current Source Delay"=w674) -> (w681:T17)
      }
      frame "Test: Check Sequence Size" {
        # "Checks Sequence step count"
        n285 = Unbundle By Name(w690) -> ("Load Current Waveform"=w694:dbl[])
        n286 = Empty Array?(array=w694) -> (empty?=w689:bool)
        n287 = case "Sequence Empty?" shown="True" w689 {
          tunnel: [w696 w698] -> w693
          tunnel: w692 -> [w696 w697]
          frame False {
          }
          frame True {
            # "Throw error"
            n288 = call "Error 6004.vi"("error in (no error)"=w697) -> ("error out"=w698:errorcluster)  [unwired: 14 in]
          }
        }
        n289 = Bundle By Name(cluster=w690, "Sequence Empty?"=w689) -> (w691:T17)
      }
      frame "Test: Check Buffer and on-board Size" {
        n290 = Unbundle By Name(w708) -> ("Sequence Empty?"=w699:bool, "Test Pins.Set Load Current"=w700:string, "Load Current Waveform"=w710:dbl[], "Test Inputs.Delay - t1 in s"=w705:dbl, "Test Inputs.Delay - t2 in s"=w704:dbl, "Test Inputs.Duration of the pulse in Second"=w703:dbl, "Test Pins.Measure Output Voltage"=w701:string)
        n291 = case shown="False" w699 {
          tunnel: w710 -> [w731 _]
          tunnel: [w728 w742] -> w707
          tunnel: w706 -> [w726 w742]
          tunnel: w705 -> [w723 _]
          tunnel: w704 -> [w722 _]
          tunnel: w703 -> [w721 _]
          tunnel: [w716 _] -> w702
          tunnel: w701 -> [w713 _]
          tunnel: w700 -> [w712 _]
          frame False {
            # "Check for memory only if sequence is valid"
            n292 = Array Size(array=w731) -> (size(s)=w730:i32)
            n293 = Compound Arithmetic op=ADD(w723, w722, w721) -> (w718:dbl)
            n294 = call "Check Scope on-board memory.vi"("Scope"=w713, "Acquisition Time"=w718, "error in (no error)"=w726) -> ("IVI Refnum out"=w720:refnum<k15>, "Required Record Length"=w719:i32, "Maximum Record Length"=w717:i32, "Insufficient Memory?"=w715:bool, "error out"=w725:errorcluster)  [unwired: 8 in]
            n295 = call "Get SMU Buffer Size.vi"("SMU"=w712, "No. of steps"=w730, "error in (no error)"=w725) -> ("Required Buffer Size"=w727:i32, "Maximum Buffer Size"=w724:i32, "Insufficient Memory"=w714:bool, "error out"=w729:errorcluster)  [unwired: 9 in]
            n296 = Or(x=w715, y=w714) -> (x .or. y?=w716:bool)
            n297 = case shown="False" w716 {
              tunnel: w729 -> [w735 w741]
              tunnel: [w734 w740] -> w728
              tunnel: w727 -> [_ w739]
              tunnel: w724 -> [_ w738]
              tunnel: w720 -> [w733 _]
              tunnel: w719 -> [w732 w737]
              tunnel: w717 -> [_ w736]
              frame False {
                # "Valid memory"
                n298 = property class="niScope"(reference=w733, error in=w735, "Min Number of Points"=w732) -> (error out=w734:errorcluster)  [unwired: 1 out]
              }
              frame True {
                # "Show error"
                n299 = call "Error 6003.vi"("Required Buffer Size"=w739, "Maximum Buffer Size"=w738, "Requested Record Length"=w737, "Maximum Record Length"=w736, "error in (no error)"=w741) -> ("error out"=w740:errorcluster)  [unwired: 10 in]
              }
            }
          }
          frame True {
          }
        }
        n300 = Bundle By Name(cluster=w708, "Insufficient memory?"=w702) -> (w709:T17)
      }
      frame "Test: Set Input Voltage" {
        n301 = call "Progress Monitor.vi"("State"=w746) -> ("State Array Index"=w749:i32)  [unwired: 14 in]
        n302 = property on="Progress" class="Slide (strict)"(error in=w747, "Value"=w749) -> (error out=w748:errorcluster)  [unwired: 1 in, 1 out]
        n303 = Unbundle By Name(w750) -> ("Test Pins.Set Input Voltage"=w743:string, "Test Inputs.Input Voltage in V"=w744:dbl)
        n304 = call "Set Source.vi"("Set Vin"=w743, "Vin in V"=w744, "error in (no error)"=w748) -> ("error out"=w745:errorcluster)  [unwired: 12 in]
      }
      frame "Test: Calc Min Delay for Max. Ref Position" {
        n305 = call "Progress Monitor.vi"("State"=w755) -> ("State Array Index"=w758:i32)  [unwired: 14 in]
        n306 = property on="Progress" class="Slide (strict)"(error in=w756, "Value"=w758) -> (error out=w757:errorcluster)  [unwired: 1 in, 1 out]
        n307 = Unbundle By Name(w759) -> ("Sequence Empty?"=w754:bool, "Insufficient memory?"=w753:bool, "Test Pins.Measure Output Voltage"=w762:string)
        n308 = Or(x=w754, y=w753) -> (x .or. y?=w752:bool)
        n309 = case shown="False" w752 {
          tunnel: [w782 w783] -> w763
          tunnel: w762 -> [w781 _]
          tunnel: [w780 _] -> w761
          tunnel: w757 -> [w779 w783]
          frame False {
            # "Reference Position % of Total Aqusition Time"
            # "in milliseconds"
            # "Total Acquisition Time"
            # "Sufficient Buffer and on-board memory and has valid sequence"
            n310 = call "Pin Name to Reference.vim"("Pin Name"=w781, "type"=refnum<k15> refnum ("instrument handle"), "error in (no error)"=w779) -> ("Reference"=w776:refnum<k15>, "error out"=w777:errorcluster)  [unwired: 7 in, 4 out]
            n311 = property class="niScope"(reference=w776, error in=w777) -> (error out=w782:errorcluster, "Reference Position"=w765:dbl, "Min Number of Points"=w766:i32, "Actual Sample Rate"=w775:dbl)  [unwired: 1 out]
            n312 = Reciprocal(x=w775) -> (1/x=w774:dbl)
            n313 = To Double Precision Float(number=w766) -> (double precision float=w773:dbl)
            n314 = Multiply(x=w773, y=w774) -> (x*y=w772:dbl)
            n315 = Divide(x=w765, y=100.0) -> (x/y=w771:dbl)
            n316 = Multiply(x=w771, y=w772) -> (x*y=w769:dbl)
            n317 = Multiply(x=w769, y=1000.0) -> (x*y=w767:dbl)
            n318 = To Unsigned Long Integer(number=w767) -> (unsigned 32bit integer=w780:u32)
          }
          frame True {
            # "Insufficient buffer and on-board memory"
          }
        }
        n319 = Bundle By Name(cluster=w759, "Min delay for Reference Position"=w761) -> (w760:T17)
      }
      frame "Test: Generate Load Current Sequence" {
        n320 = Unbundle By Name(w798) -> ("Sequence name"=w788:string, "Load Current Source Delay"=w791:dbl[], "Load Current Waveform"=w789:dbl[], "Test Pins.Set Load Current"=w792:string, "Min delay for Reference Position"=w787:u32, "Test Pins.Measure Output Voltage"=w793:string, "Insufficient memory?"=w786:bool, "Sequence Empty?"=w784:bool)
        n321 = call "Progress Monitor.vi"("State"=w795) -> ("State Array Index"=w797:i32)  [unwired: 14 in]
        n322 = property on="Progress" class="Slide (strict)"(error in=w796, "Value"=w797) -> (error out=w794:errorcluster)  [unwired: 1 in, 1 out]
        n323 = Or(x=w786, y=w784) -> (x .or. y?=w785:bool)
        n324 = case shown="False" w785 {
          tunnel: w794 -> [w815 w817]
          tunnel: w793 -> [w814 _]
          tunnel: w792 -> [w810 _]
          tunnel: w791 -> [w807 _]
          tunnel: [w804 w817] -> w790
          tunnel: w789 -> [w803 _]
          tunnel: w788 -> [w802 _]
          tunnel: w787 -> [w800 _]
          frame False {
            # "Sufficient buffer and on-board memory and has valid sequence"
            n325 = call "Pin Name to Reference.vim"("Pin Name"=w814, "type"=refnum<k15> refnum ("instrument handle"), "error in (no error)"=w815) -> ("Reference"=w812:refnum<k15>, "error out"=w813:errorcluster)  [unwired: 7 in, 4 out]
            n326 = Add Array Elements(numeric array=w807) -> (sum=w805:dbl)
            n327 = call <instrlib>:"niScope Initiate Acquisition.vi"("instrument handle"=w812, "error in"=w813) -> ("error out"=w806:errorcluster)  [unwired: 12 in, 1 out]
            n328 = call "Stall Data Flow.vim"("value in"=w806, "milliseconds to wait"=w800) -> ("value out"=w801:errorcluster)  [unwired: 1 out]
            n329 = call "Pin Name to Reference.vim"("Pin Name"=w810, "type"=refnum<k15> refnum ("instrument handle"), "error in (no error)"=w801) -> ("Reference"=w811:refnum<k15>, "error out"=w809:errorcluster)  [unwired: 7 in, 4 out]
            n330 = call "Generate load Current Sequence.vi"("Load SMU Reference"=w811, "sequence name"=w802, "Total Aquisition Time (s)"=w805, "Load Current Sequence"=w803, "error in (no error)"=w809) -> ("error out"=w804:errorcluster)  [unwired: 9 in, 1 out]
          }
          frame True {
            # "Insufficient buffer and on-board memory"
          }
        }
      }
      frame "Test: Measure Transient" {
        n331 = Unbundle By Name(w837) -> ("Sequence Empty?"=w821:bool, "Insufficient memory?"=w818:bool, "Current Measurement Option"=w826:T16, "Load Current Waveform"=w827:dbl[], "Test Pins.Measure Load Current"=w825:string, "Load Current Source Delay"=w832:dbl[], "Test Inputs.Shunt Resistance (Ohm)"=w824:dbl, "Test Pins.Measure Output Voltage"=w833:string, "Scope Channels"=w822:string, "Test Inputs.Advance Setting.Prepare.Load SMU Record Length"=w820:i32)
        n332 = call "Progress Monitor.vi"("State"=w834) -> ("State Array Index"=w836:i32)  [unwired: 14 in]
        n333 = property on="Progress" class="Slide (strict)"(error in=w835, "Value"=w836) -> (error out=w823:errorcluster)  [unwired: 1 in, 1 out]
        n334 = Or(x=w821, y=w818) -> (x .or. y?=w819:bool)
        n335 = case shown="False" w819 {
          tunnel: w833 -> [w864 _]
          tunnel: w832 -> [w861 _]
          tunnel: [w840 _] -> w831
          tunnel: [w860 _] -> w830
          tunnel: [w853 w866] -> w829
          tunnel: [w841 _] -> w828
          tunnel: w827 -> [w851 _]
          tunnel: w826 -> [w850 _]
          tunnel: w825 -> [w849 _]
          tunnel: w824 -> [w848 _]
          tunnel: w823 -> [w846 w866]
          tunnel: w822 -> [w842 _]
          tunnel: w820 -> [_ _]
          frame False {
            # "5 multiples to have enough timeout"
            # "sufficient buffer and on-board memory and has valid sequence"
            n336 = call "Pin Name to Reference.vim"("Pin Name"=w864, "type"=refnum<k15> refnum ("instrument handle"), "error in (no error)"=w846) -> ("Reference"=w863:refnum<k15>, "error out"=w845:errorcluster)  [unwired: 7 in, 4 out]
            n337 = property class="niScope"(reference=w863, error in=w845) -> (reference out=w862:refnum<k15>, error out=w855:errorcluster, "Trigger Delay"=w843:dbl, "Actual Record Length"=w844:i32, "Actual Sample Rate"=w860:dbl)
            n338 = Add Array Elements(numeric array=w861) -> (sum=w852:dbl)
            n339 = To Double Precision Float(number=w844) -> (double precision float=w859:dbl)
            n340 = Divide(x=w859, y=w860) -> (x/y=w858:dbl)
            n341 = Multiply(x=5.0, y=w858) -> (x*y=w856:dbl)
            n342 = call "Scope Measurement.vi"("Scope Reference"=w862, "Scope Channels"=w842, "error in (no error)"=w855, "Scope Timeout (s)"=w856) -> ("Measured Output Voltage"=w841:cluster{dbl[], dbl[]}, "Measured Load Current"=w847:cluster{dbl[], dbl[]}, "error out"=w854:errorcluster)  [unwired: 9 in]
            n343 = call "Current Measurement.vi"("Cature Load Currrent Pin Name"=w849, "Load Current Sequence"=w851, "Enum"=w850, "Total Aquisition Time (s)"=w852, "Shunt Resistance"=w848, "Measured Scope Load Current"=w847, "error in (no error)"=w854, "Trigger Delay"=w843) -> ("Measured Load Current"=w840:cluster{"x-axis":dbl[], "wfm":dbl[]}, "error out"=w853:errorcluster)  [unwired: 6 in]
          }
          frame True {
            # "Insufficient buffer and on-board memory"
          }
        }
        n344 = Bundle By Name(cluster=w837, "Test Results.Measured Output Voltage"=w828, "Test Results.Measured Load Current"=w831, "Test Results.Actual Sample Rate in S/s"=w830) -> (w838:T17)
      }
      frame "Test: Calculate Out. Voltage Threshold" {
        # "Calculate reference Voltage Level for Settling time"
        n345 = call "Progress Monitor.vi"("State"=w867) -> ("State Array Index"=w870:i32)  [unwired: 14 in]
        n346 = property on="Progress" class="Slide (strict)"(error in=w868, "Value"=w870) -> (error out=w869:errorcluster)  [unwired: 1 in, 1 out]
        n347 = Unbundle By Name(w871) -> ("Test Inputs.Settling Time Calc Option"=w877:T11, "Test Inputs.Ref Voltage level for Settling Time Calc"=w876:dbl, "Test Inputs.% of Vnom for Settling Time Calc"=w875:dbl, "Test Inputs.Nominal Output Voltage in V"=w874:dbl)
        n348 = case shown="\"Voltage Level \", Default" w877 {
          tunnel: w876 -> [w879 _]
          tunnel: w875 -> [_ w881]
          tunnel: w874 -> [_ w882]
          tunnel: [w879 w880] -> w873
          frame "Voltage Level ", Default {
          }
          frame "Percentage of Vnom" {
            n349 = formula code="y = (x/100)*v;"("x"=w881, "v"=w882) -> ("y"=w880:dbl)
          }
        }
        n350 = Bundle By Name(cluster=w871, "Test Inputs.Ref Voltage level for Settling Time Calc"=w873) -> (w872:T17)
      }
      frame "Test: Calculate Settling Time" {
        n351 = call "Progress Monitor.vi"("State"=w883) -> ("State Array Index"=w886:i32)  [unwired: 14 in]
        n352 = Unbundle By Name(w887) -> ("Output Voltage Coupling"=w889:i32, "Test Results.Measured Output Voltage.wfm"=w896:dbl[], "Test Inputs.Ref Voltage level for Settling Time Calc"=w895:dbl, "Test Inputs.Duration of the pulse in Second"=w894:dbl, "Test Results.Actual Sample Rate in S/s"=w893:dbl, "Test Inputs.Nominal Output Voltage in V"=w890:dbl)
        n353 = property on="Progress" class="Slide (strict)"(error in=w884, "Value"=w886) -> (error out=w885:errorcluster)  [unwired: 1 in, 1 out]
        n354 = call "CalculateSettlingTime.vi"("Waveform"=w896, "Waveform Coupling"=w889, "Recovery Volt Level (V)"=w895, "Duration of the pulse (s)"=w894, "Sampling Freq (S/s)"=w893, "DC Component (v)"=w890) -> ("FirstSpike. Duration (s)"=w892:dbl, "SecondSpike. Duration (s)"=w891:dbl)  [unwired: 8 in]
        n355 = Bundle By Name(cluster=w887, "Test Results.First Edge - Settling Time in s"=w892, "Test Results.Second Edge - Settling Time in s"=w891) -> (w888:T17)
      }
      frame "Test: Cleanup DCPower" {
        w902 = 1026 items=["Automatically after Source Complete"=1025, "On Demand"=1026, "On Measure Trigger"=1027] ("Measurement:Advanced:Measure When")
        w924 = T24 1020 items=["Single Point"=1020, "Sequence"=1021] ("source mode")
        w927 = T23 1006 items=["DC Voltage"=1006, "DC Current"=1007, "Pulse Voltage"=1049, "Pulse Current"=1050] ("output function")
        # "Setting to default"
        # "Adding abort here \nsince sequence cannot be ended while running"
        # "Set Single point Voltage mode as default"
        n356 = Unbundle By Name(w936) -> ("Test Pins.Set Input Voltage"=w932:string, "Insufficient memory?"=w899:bool, "Sequence Empty?"=w900:bool, "Sequence name"=w921:string, "Test Pins.Set Load Current"=w934:string)
        n357 = call "Progress Monitor.vi"("State"=w928) -> ("State Array Index"=w931:i32)  [unwired: 14 in]
        n358 = property on="Progress" class="Slide (strict)"(error in=w929, "Value"=w931) -> (error out=w930:errorcluster)  [unwired: 1 in, 1 out]
        n359 = call "Pin Name to Reference.vim"("Pin Name"=w934, "type"=refnum<k15> refnum ("instrument handle"), "error in (no error)"=w930) -> ("Reference"=w913:refnum<k15>, "error out"=w914:errorcluster)  [unwired: 7 in, 4 out]
        n360 = Or(x=w899, y=w900) -> (x .or. y?=w898:bool)
        n361 = call <instrlib>:"niDCPower Abort.vi"("error in (no error)"=w914, "instrument handle"=w913) -> ("error out"=w922:errorcluster, "instrument handle out"=w923:refnum<k15>)  [unwired: 8 in]
        n362 = case shown="False" w898 {
          tunnel: w923 -> [w945 w946]
          tunnel: w922 -> [w944 w947]
          tunnel: w921 -> [w940 _]
          tunnel: [w939 w947] -> w912
          tunnel: [w938 w946] -> w909
          frame False {
            # "Sequence should be empty to enable\\disable output"
            # "Sequence available"
            n363 = call <instrlib>:"niDCPower Delete Advanced Sequence With Channels.vi"("error in (no error)"=w944, "sequence name"=w940, "instrument handle"=w945) -> ("error out"=w943:errorcluster, "instrument handle out"=w942:refnum<k15>)  [unwired: 7 in]
            n364 = property class="niDCPower"(reference=w942, error in=w943, "Active Advanced Sequence"="") -> (reference out=w938:refnum<k15>, error out=w939:errorcluster)
          }
          frame True {
            # "Sequence not created"
          }
        }
        n365 = call <instrlib>:"niDCPower Configure Output Enabled.vi"("error in (no error)"=w912, "output enabled"=FALSE, "instrument handle"=w909) -> ("error out"=w910:errorcluster, "instrument handle out"=w906:refnum<k15>)  [unwired: 7 in]
        n366 = call <instrlib>:"niDCPower Abort With Channels.vi"("error in (no error)"=w910, "instrument handle"=w906) -> ("error out"=w907:errorcluster, "instrument handle out"=w905:refnum<k15>)  [unwired: 8 in]
        n367 = call <instrlib>:"niDCPower Configure Source Mode With Channels.vi"("error in (no error)"=w907, "source mode"=w924, "instrument handle"=w905) -> ("error out"=w926:errorcluster, "instrument handle out"=w925:refnum<k15>)  [unwired: 7 in]
        n368 = call <instrlib>:"niDCPower Configure Output Function.vi"("error in (no error)"=w926, "output function"=w927, "instrument handle"=w925) -> ("error out"=w911:errorcluster, "instrument handle out"=w903:refnum<k15>)  [unwired: 7 in]
        n369 = property class="niDCPower"(reference=w903, error in=w911, "Measure Record Length"=1 ("Measurement:Measure Record Length"), "Measure When"=w902) -> (error out=w904:errorcluster)  [unwired: 1 out]
        n370 = call "Pin Name to Reference.vim"("Pin Name"=w932, "type"=refnum<k15> refnum ("instrument handle"), "error in (no error)"=w904) -> ("Reference"=w918:refnum<k15>, "error out"=w919:errorcluster)  [unwired: 7 in, 4 out]
        n371 = call <instrlib>:"niDCPower Configure Output Enabled.vi"("error in (no error)"=w919, "output enabled"=FALSE, "instrument handle"=w918) -> ("error out"=w917:errorcluster, "instrument handle out"=w916:refnum<k15>)  [unwired: 7 in]
        n372 = call <instrlib>:"niDCPower Abort With Channels.vi"("error in (no error)"=w917, "instrument handle"=w916) -> ("error out"=w915:errorcluster)  [unwired: 8 in, 1 out]
      }
      frame "Test: Cleanup Scope" {
        w948 = FALSE
        n373 = call "Progress Monitor.vi"("State"=w955) -> ("State Array Index"=w958:i32)  [unwired: 14 in]
        n374 = property on="Progress" class="Slide (strict)"(error in=w956, "Value"=w958) -> (error out=w957:errorcluster)  [unwired: 1 in, 1 out]
        n375 = Unbundle By Name(w961) -> ("Current Measurement Option"=w950:T16, "Test Pins.Measure Load Current"=w949:string, "Test Pins.Measure Output Voltage"=w960:string)
        n376 = call "Pin Name to Reference.vim"("Pin Name"=w960, "type"=refnum<k15> refnum ("instrument handle"), "error in (no error)"=w957) -> ("Reference"=w963:refnum<k15>, "Channel"=w962:string, "error out"=w964:errorcluster)  [unwired: 7 in, 3 out]
        n377 = property class="niScope"(reference=w963, error in=w964, "Active Channel"=w962, "Channel Enabled"=w948) -> (reference out=w953:refnum<k15>, error out=w951:errorcluster)
        n378 = case shown="\"Scope Measurement\"" w950 {
          tunnel: [w967 w977] -> w954
          tunnel: w953 -> [_ w977]
          tunnel: [w971 w976] -> w952
          tunnel: w951 -> [w970 w976]
          tunnel: w949 -> [w969 _]
          tunnel: w948 -> [w968 _]
          frame "Scope Measurement" {
            # "Enable/ Disable if this channel is\nselected for current measurement"
            n379 = call "Pin Name to Reference.vim"("Pin Name"=w969, "type"=refnum<k15> refnum ("instrument handle"), "error in (no error)"=w970) -> ("Reference"=w973:refnum<k15>, "Channel"=w972:string, "error out"=w974:errorcluster)  [unwired: 7 in, 3 out]
            n380 = property class="niScope"(reference=w973, error in=w974, "Active Channel"=w972, "Channel Enabled"=w968) -> (reference out=w967:refnum<k15>, error out=w971:errorcluster)
          }
          frame "SMU Measurement" {
          }
        }
        n381 = call <instrlib>:"niScope Abort.vi"("instrument handle"=w954, "error in"=w952) -> ("error out"=w959:errorcluster)  [unwired: 12 in, 1 out]
      }
      frame "Test: Update UI" {
        # "If you want to update more indicators in the front panel do it here. It is efficient to update the UI in one case rather than in several cases. Also, it is a good practice to store the results in the data cluster in an efficient format and then get the data from data cluster and update the UI, in that way we could have the front panel independent of how we manipulate the data."
        n382 = call "Progress Monitor.vi"("State"=w981) -> ("State Array Index"=w984:i32)  [unwired: 14 in]
        n383 = Unbundle By Name(w988) -> ("Test Results.Measured Output Voltage"=w980:cluster{"x-axis":dbl[], "wfm":dbl[]}, "Test Results.Measured Load Current"=w978:cluster{"x-axis":dbl[], "wfm":dbl[]}, "Test Results"=→"Test Results":T14, "Test Results.First Edge - Settling Time in s"=→"First Edge - Settling Time (s)":dbl, "Test Results.Second Edge - Settling Time in s"=→"Second Edge - Settling Time (s)":dbl)
        n384 = property on="Progress" class="Slide (strict)"(error in=w982, "Value"=w984) -> (error out=w983:errorcluster)  [unwired: 1 in, 1 out]
        n385 = Build Array(w980, w978) -> (→"Load Transient":cluster{"x-axis":dbl[], "wfm":dbl[]}[])
      }
      frame "Test: End" {
        # "End of the Test Procedure. Do cleanup of resources or references."
        n386 = call "Progress Monitor.vi"("State"=w990) -> ("State Array Index"=w993:i32)  [unwired: 14 in]
        n387 = property on="Progress" class="Slide (strict)"(error in=w991, "Value"=w993) -> (error out=w992:errorcluster)  [unwired: 1 in, 1 out]
      }
      frame "---------------------Misc-----------------------" {
      }
      frame "Error" {
        # "Handle the error and make sure to clear the error."
        n388 = Unbundle By Name(w1002) -> ("Termination Monitor Info.Caller Information.Mode"=w1001:T8)
        n389 = case shown="\"MeasurementSuite\"" w1001 {
          tunnel: w1005 -> [w1009 w1014 w1016]
          tunnel: [w1007 w1011 w1015] -> w1003
          tunnel: [_ TRUE _] -> w1000
          tunnel: w999 -> [_ w1012 _]
          frame "Standalone" {
            w1006 = T25 2 items=["no dialog", "OK message", "continue or stop message", "OK message + warnings", "continue/stop + warnings"] ("type of dialog (OK msg:1)")
            n390 = call <vilib>:"General Error Handler.vi"("type of dialog (OK msg:1)"=w1006, "error in (no error)"=w1009) -> ("error out"=w1008:errorcluster)  [unwired: 9 in, 4 out]
            n391 = call <vilib>:"Clear Errors.vi"("error in (no error)"=w1008) -> ("error out"=w1007:errorcluster)  [unwired: 5 in, 1 out]
          }
          frame "Automation" {
            n392 = call <userlib>:"Release.vi"("Queue in"=w1012) -> ("Error Out"=w1010:errorcluster)  [unwired: 14 in]
            n393 = Merge Errors(w1014, w1010) -> (w1011:errorcluster)
          }
          frame "MeasurementSuite" {
            n394 = property on="ErrorOccured" class="Clust (strict)"("Val(Sgnl)"=w1016) -> (error out=w1015:errorcluster)  [unwired: 2 in, 1 out]
          }
        }
      }
      frame "Exit" {
        # "Last case called before stopping the execution. \nError occured in this state will not be captured by Error state."
        n395 = call <userlib>:"Release.vi"("Queue in"=w1022, "Error In"=w1023) -> ("Error Out"=w1018:errorcluster)  [unwired: 13 in]
        n396 = property on="Progress" class="Slide (strict)"(error in=w1018, "Visible"=FALSE) -> (error out=w1017:errorcluster)  [unwired: 1 in, 1 out]
      }
    }
  }
  "error out" <- w4
  "Header" <- "Load Transient" ("Header")
